vi "VRE17.vi"() -> ()   [LabVIEW 2012]
uses:
  <vilib>/userdefined/High Color/IMAQdx.ctl
  <vilib>/addons/Machine Learning/Utilities/Riffle (cluster).vi
  <vilib>/Analysis/baseanly.llb/Unimode.vi
  <vilib>/Analysis/baseanly.llb/Mean (DBL).vi
  <vilib>/Utility/file.llb/Write To Spreadsheet File (string).vi
  <vilib>/Utility/file.llb/Write To Spreadsheet File (DBL).vi
  <vilib>/regexp/Match Regular Expression.xnode
  <vilib>/vision/NI_Vision_Development_Module.lvlib
  <vilib>/vision/driver/NI_Vision_Acquisition_Software.lvlib
  <vilib>/Analysis/NI_AALBase.lvlib
  <vilib>/addons/Machine Learning/NILabs_MLT.lvlib
panel:
  in  "forced stop":bool
  out "Don't":bool
  out "LR invert all":bool
  in  "LR invert manual":bool
  out "moduleNum":u8
  out "moduleTime":u16
  out "nextMovieID":u8
  out "nextPerturbID":u8
  out "movieSeq":u8[](array[numeric])
  out "perturbSeq":u8[](array[numeric])
  in  "tON":u16=390
  in  "z3":u32=390
  in  "z1":u32=390
  out "moduleNumPrevious":u8
  out "moviePrimed":bool
  out "expTime":u16
  out "t0":u32
  out "movieR":u8
  out "active":i16
  out "m_buffer2":i8[](array[numeric])
  out "c_buffer 2":dbl[](array[numeric])
  out "w":dbl=50.0
  in  "Acquisition #":dbl
  in  "Basename":string
  out "sec":u16
  out "min":u16
  out "fileNumber":string
  in  "Tab Control":enum32{"User", "Manager", "protocol"}(tab)
  in  "Quiet mode":bool=TRUE
  in  "yawDrift":dbl=0.004
  in  "frdDrift":dbl=-0.002
  out "perturb wait":u16
  out "movie wait":u16
  out "perturb":u16(ring) items=["", "VR halt", "LR invert"]
  out "movie":u16(ring) items=["", "real fish", "h. ellipse", "v. ellipse", "feeding"]
  out "perturb ON":bool
  out "movie ON":bool
  out "movieID":u8
  out "perturbID":u8
  in  "LR invert":bool
  in  "yawCoef_L":dbl=1.1
  in  "yawCoef_R":dbl=1.1
  in  "keepSetting":bool
  in  "2P fps":dbl=30.0
  in  "Recording (min)":dbl=30.2
  out "2P frame":dbl
  in  "start experiment":bool
  in  "align done":bool
  out "LV loop time":u32
  in  "loop time (ms)":u32=20
  out "vreFps (ms)":dbl
  in  "frdCoef":dbl=0.25
  in  "yawIn threshold for movie":dbl=0.9
  in  "movie hijack":dbl=1.0
  in  "th1":dbl
  in  "th2":dbl
  out "m":dbl
  in  "Set baseline curv = 0 (for debug)":bool
  out "baseline curv":dbl
  in  "frdOmrVRE":bool
  in  "hijCoef2":dbl=10.0
  in  "hijCoef1":dbl=5.0
  in  "frd_hijack":dbl
  in  "yaw_hijack":i8
  in  "hijack":bool
  in  "th_darkBG":dbl=70.0
  out "blobs":dbl
  in  "decayR":dbl=0.9
  in  "cc^2":bool=TRUE
  in  "moviePrimedOff":u16=390
  in  "perturbDuration":u16=10
  in  "moviePrimedON":u16=240
  in  "perturbOnset":u16=120
  in  "modDuration":u16=450
  in  "Yres":i32=90
  in  "Xres":i32=120
  out "i":i32
  out "forward display":dbl(graph)
  in  "decayF":dbl=0.9
  out "zeroCross":i16
  out "cc":dbl
  out "m2":dbl[](array[numeric])
  out "m1":dbl[](array[numeric])
  out "I":u8[][](array[numeric])
  out "qCtr":dbl
  out "segL":dbl
  out "refine5ind":dbl[](array[numeric])
  out "xc":dbl
  out "yaw display":dbl(graph)
  out "cCurv1":dbl format="%0.2f"
  out "set 2P frames":dbl
  out "headingAngle":dbl
  out "virtual location":cluster{dbl[], dbl[]}[](graph)=[{[-0.0], [0.0]}, {[1.8369701987210297e-16], [3.0]}]
  out "trackPt":dbl[][](array[numeric])
  out "m_buffer":dbl[](array[numeric])
  out "c_buffer":dbl[](array[numeric])
  out "frdInput":dbl
  out "yawInput":dbl
  out "pix#":i32
  out "trackPt txt":path
  out "trackPt#":i32
  out "Image_save":T1(plugin-control) caption="Image"
  out "Session Out":T2
  out "data tif":refnum<file>
  in  "fx":dbl=120.0
  in  "fy":dbl=90.0
  out "par txt":path
  out "ROI":i32[](array[numeric])
  out "Bottom":i32
  out "Right":i32
  out "Top":i32
  out "Left":i32
  out "data txt":path
  out "y":dbl
  out "x":dbl
  out "forward":dbl
  out "yaw":dbl
  out "txt":dbl[][](array[numeric])
  out "txt row#":u64
  # "Right tunnel"
  # "Behavioral recording"
  # "27 min\n23 min\n18 min\n14 min\n10 min\n5 min\n1 min"
  # "Left tunnel"
  # "Set yawCoef_R & yawCoef_L so that max(yawInput) ~0.5"
  # "Set frdCoef so that max(frdInput) ~0.1"
  # "VRE update"
  # "VR perturbation"
  # "movie"
  # "VRE hijack"
  # "Define inactive frame to \nmeasure baseline curvature"
  # "Define active frames to \npermit classification"
  # "(in seconds)"
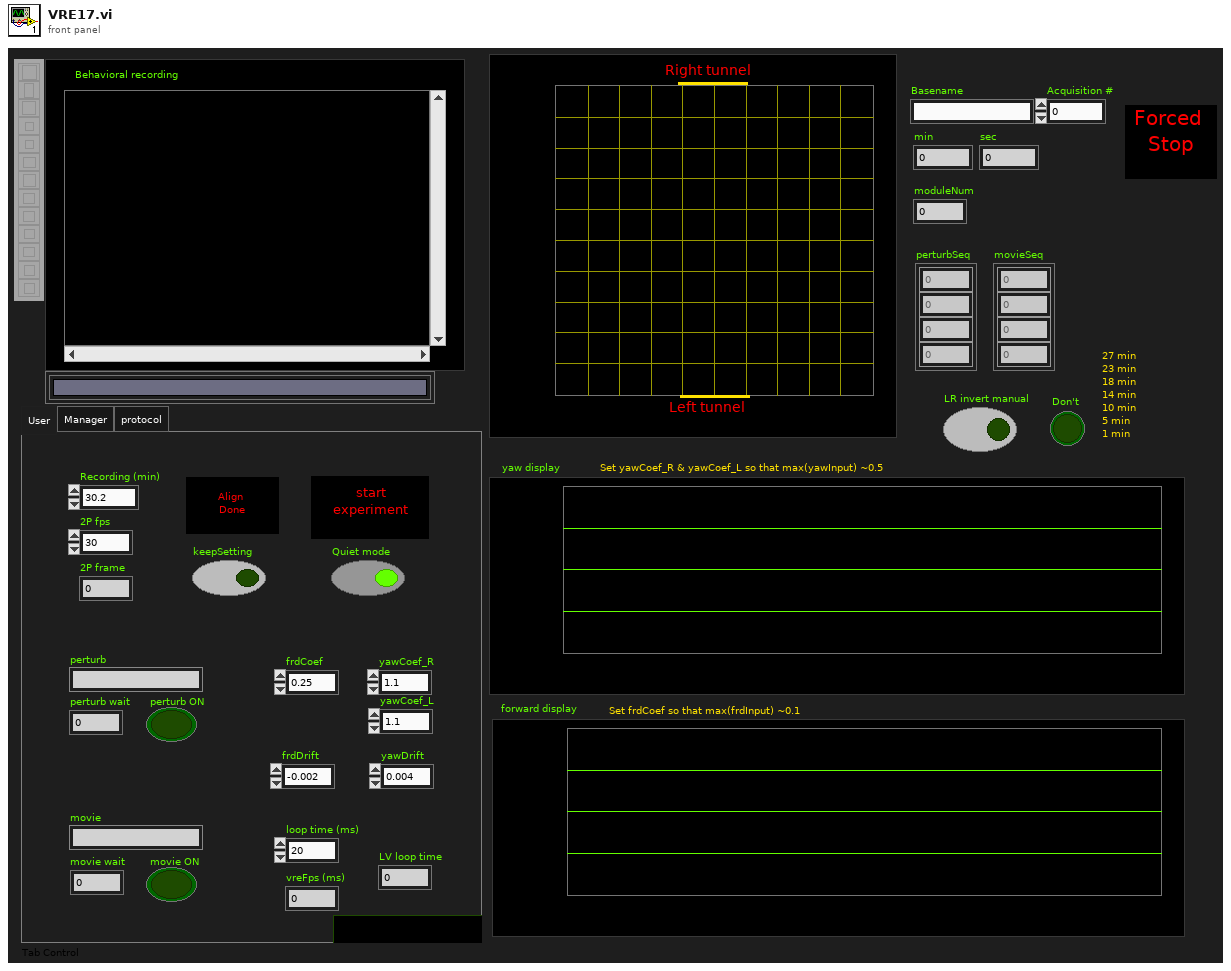
[diagram p1: front panel]
types:
  T1 = typedef "IMAQ Image.ctl" = refnum<image>
  T2 = typedef "IMAQdx.ctl" = refnum<k21>
  T3 = typedef "IMAQ Rectangle" = cluster{"Left":i32, "Top":i32, "Right":i32, "Bottom":i32, "Rotation":dbl}
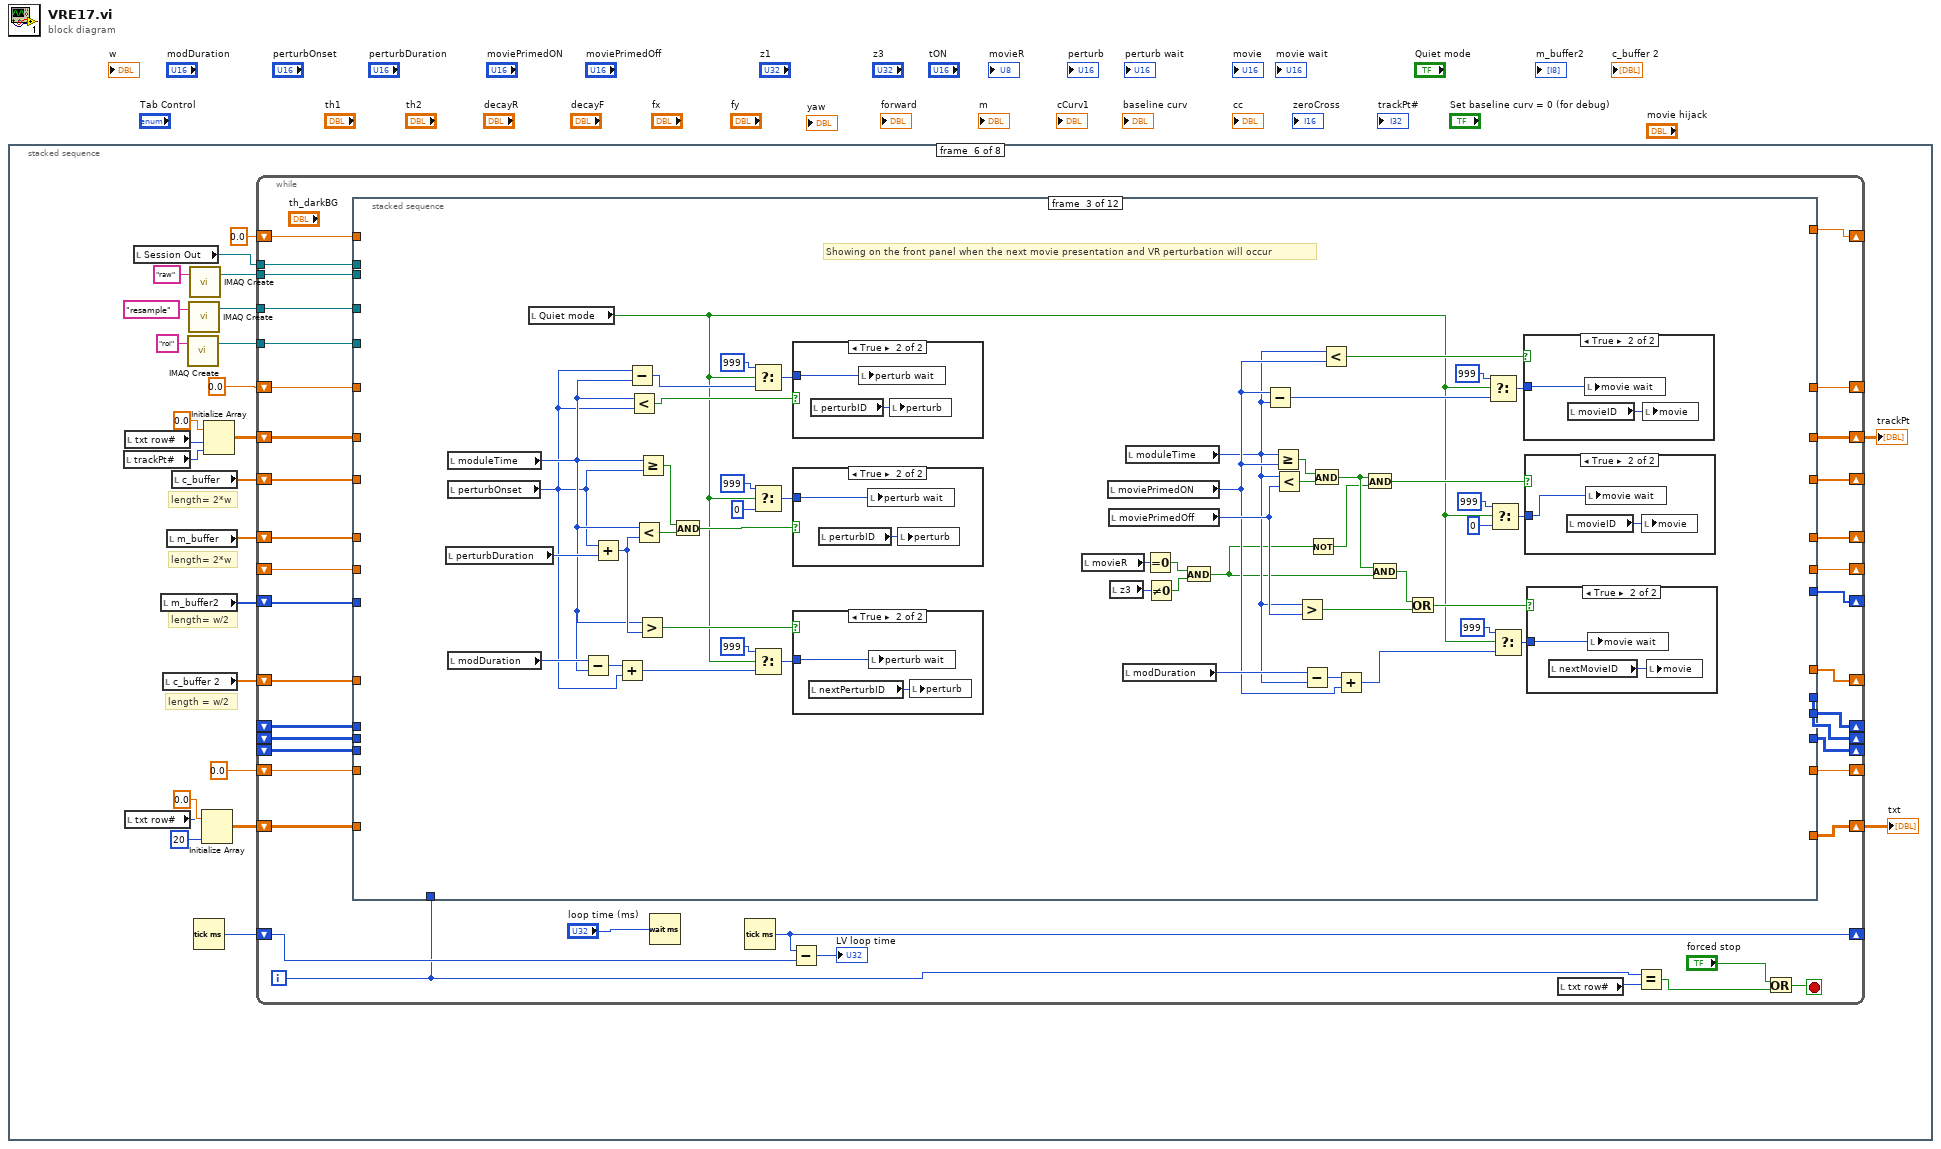
[diagram p0: block diagram]
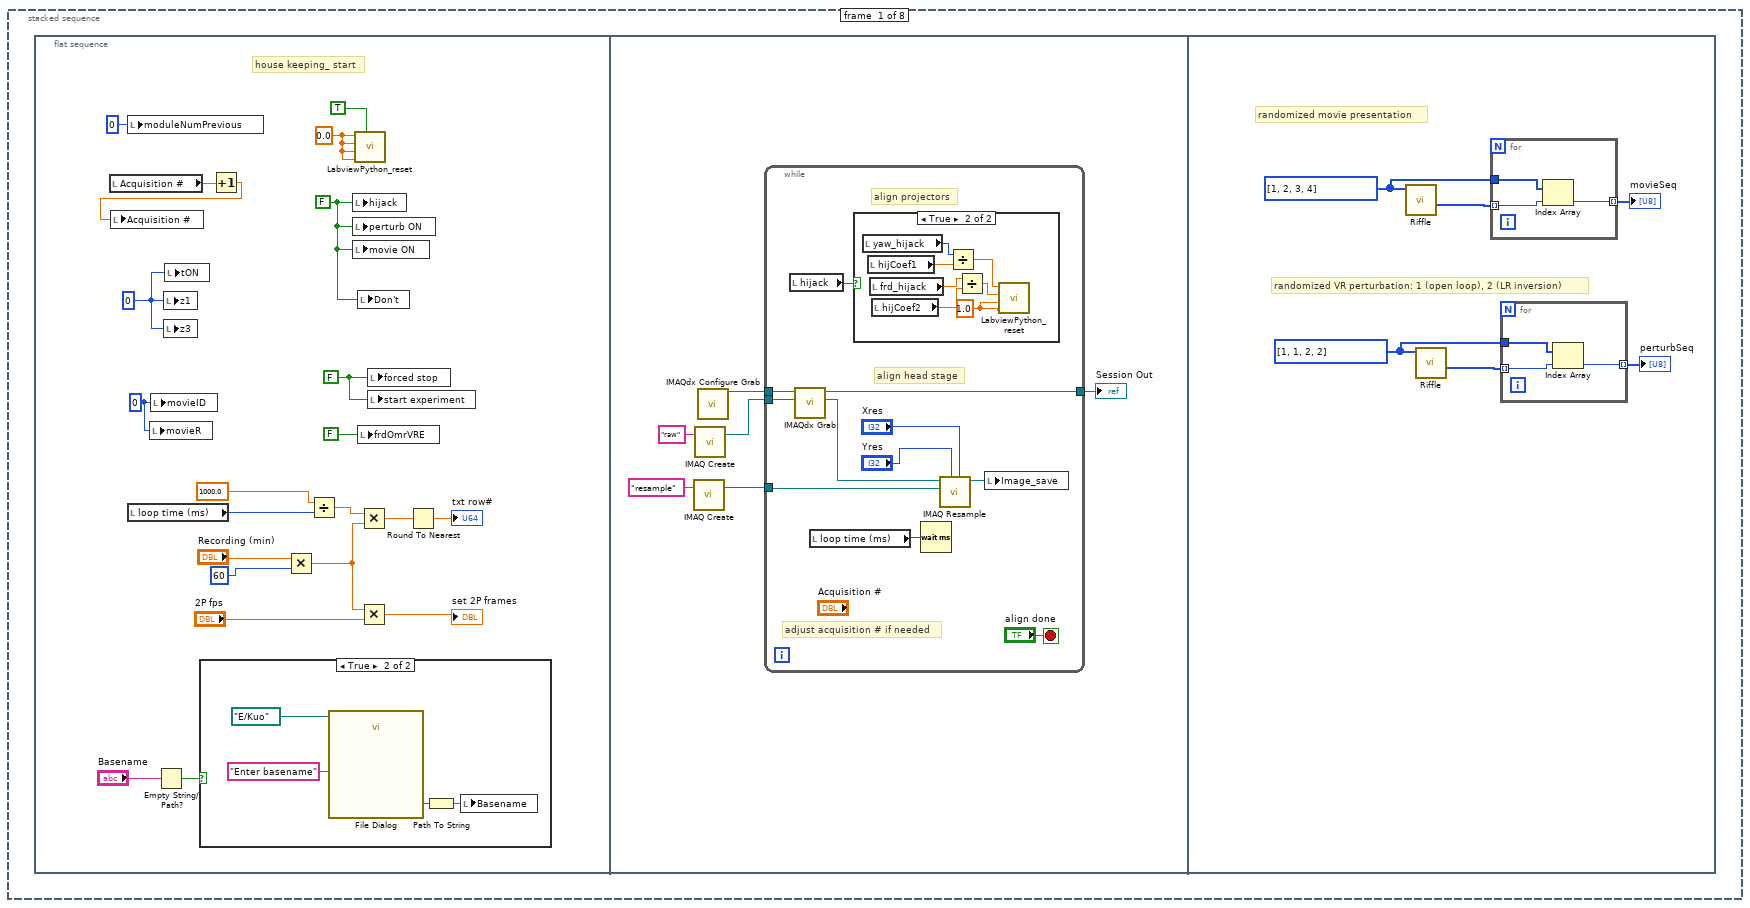
[diagram p2: hidden frame]
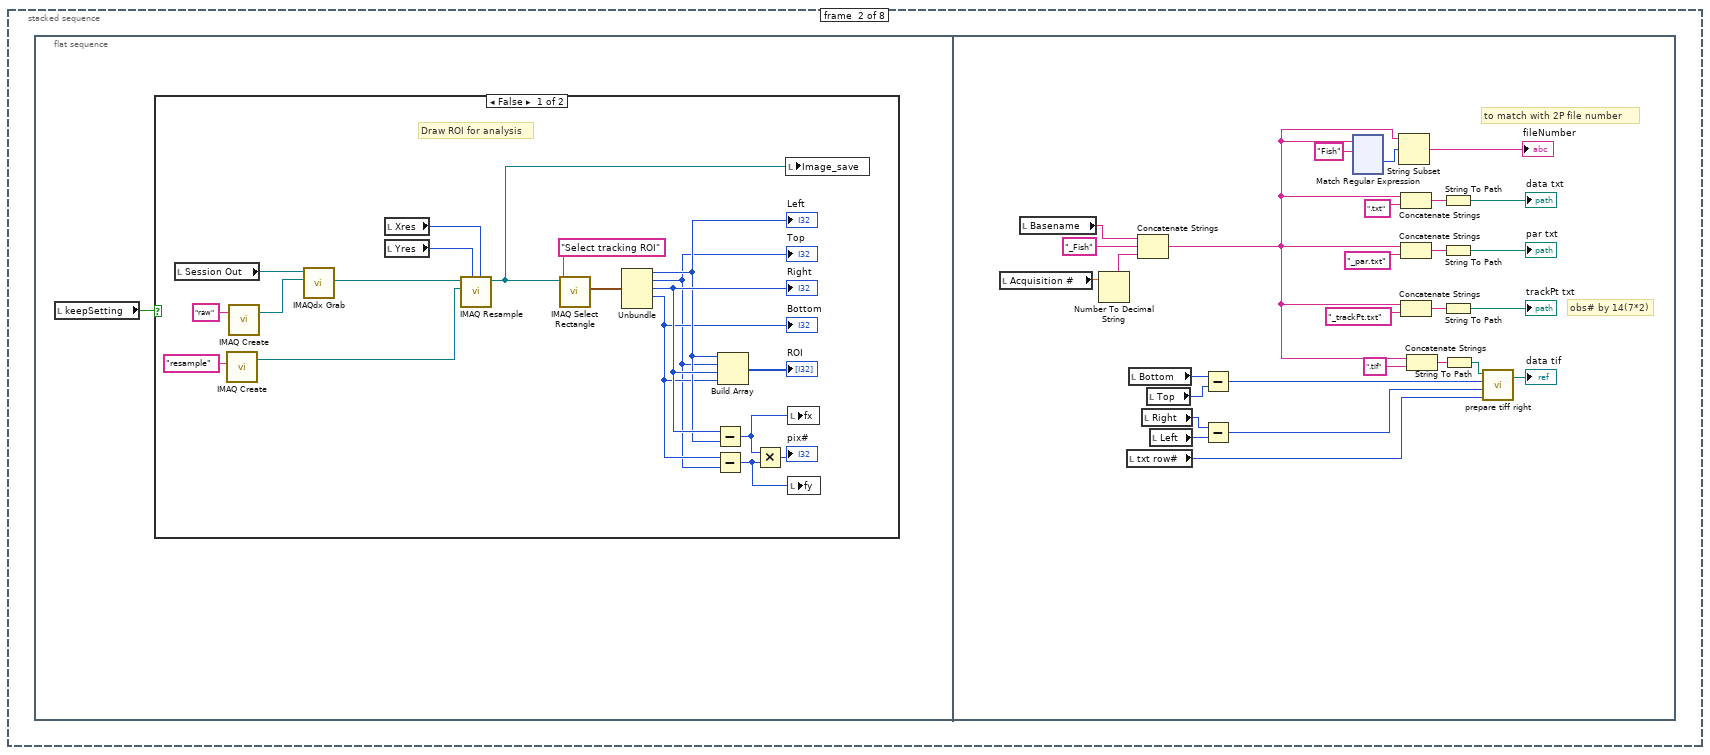
[diagram p5: hidden frame]
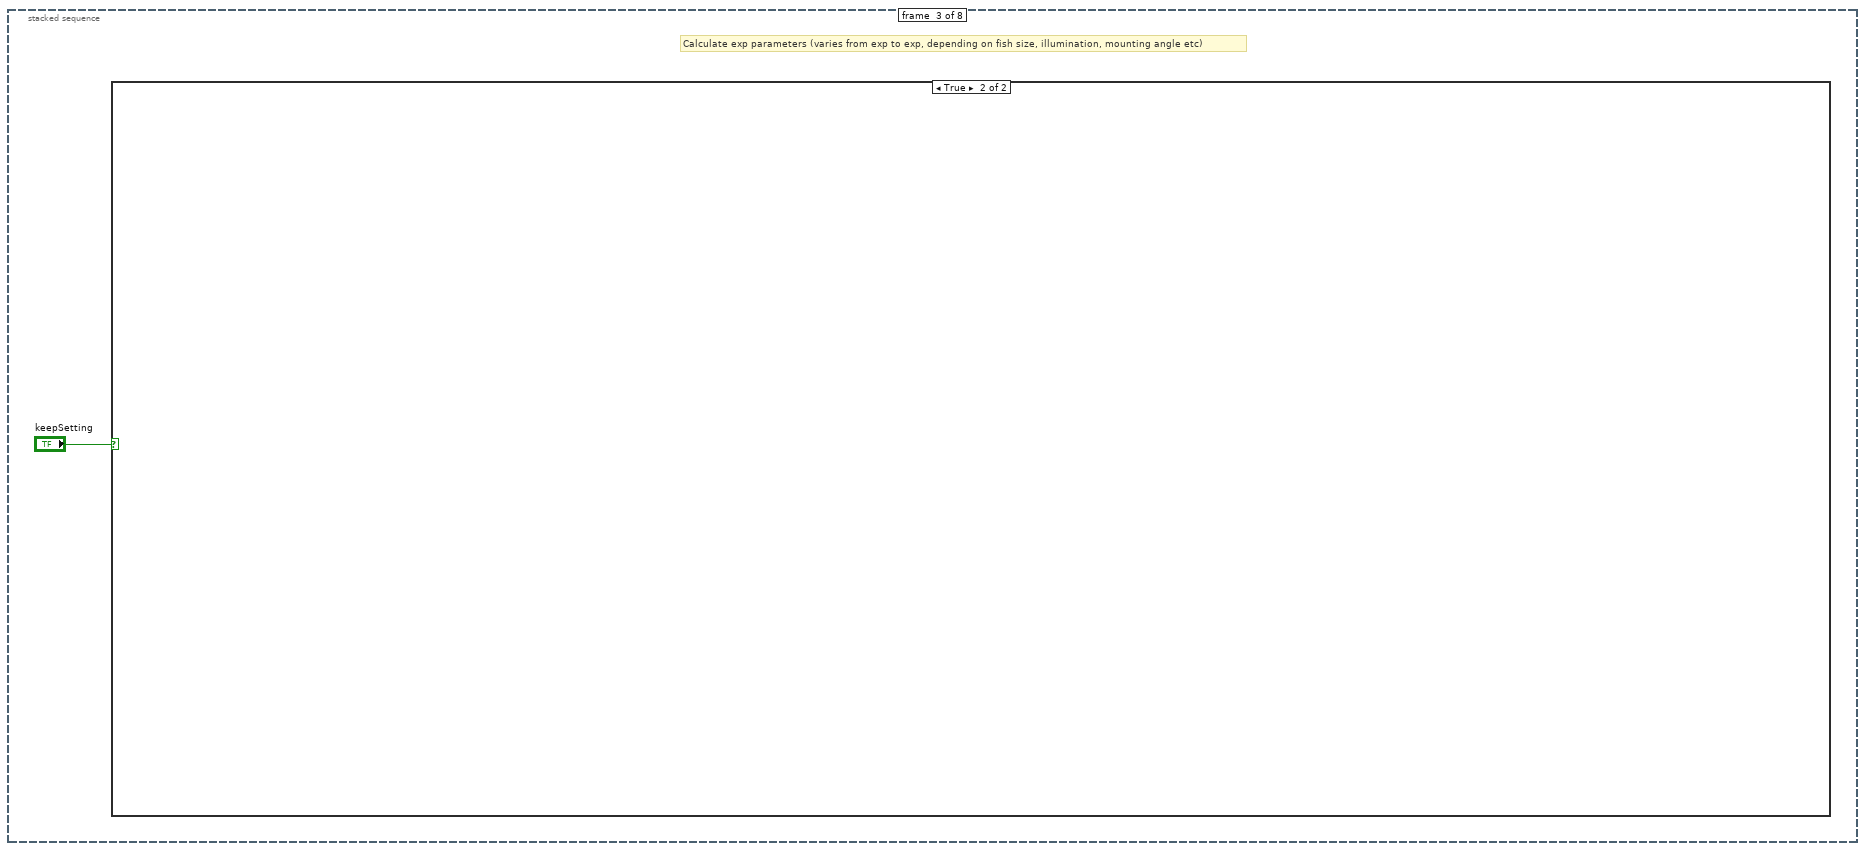
[diagram p7: hidden frame]
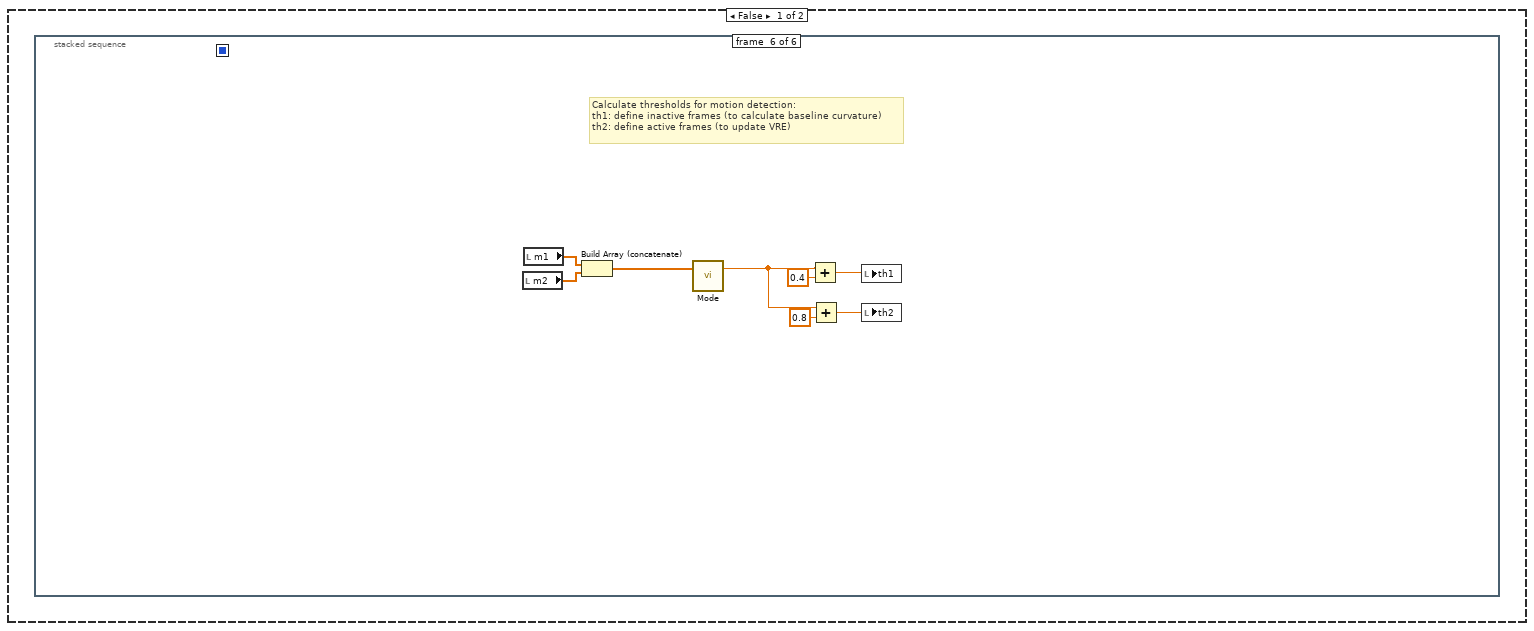
[diagram p8: hidden frame]
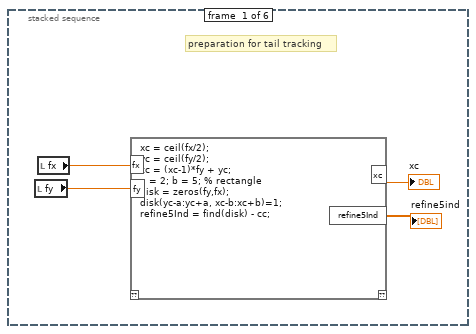
[diagram p9: hidden frame]
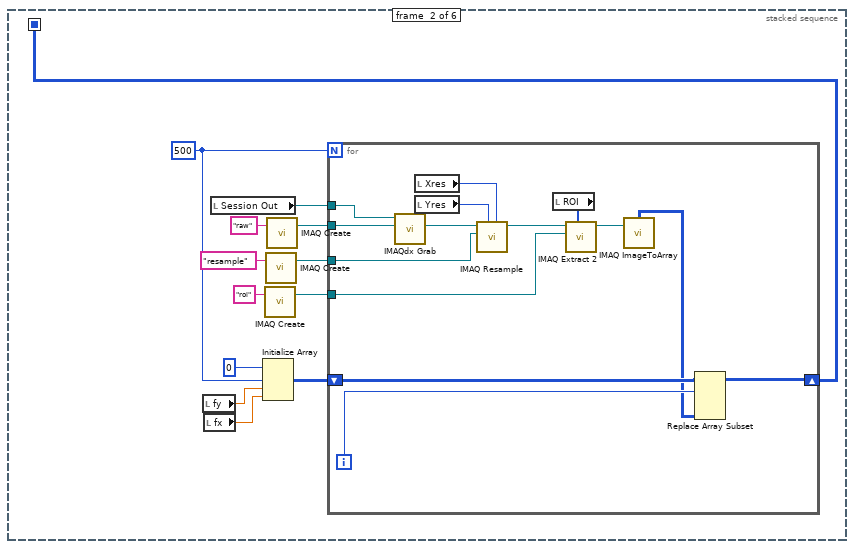
[diagram p10: hidden frame]
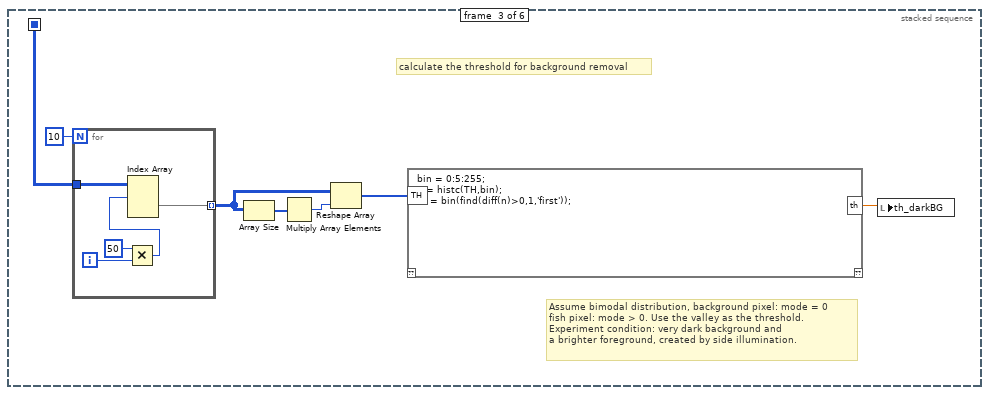
[diagram p11: hidden frame]
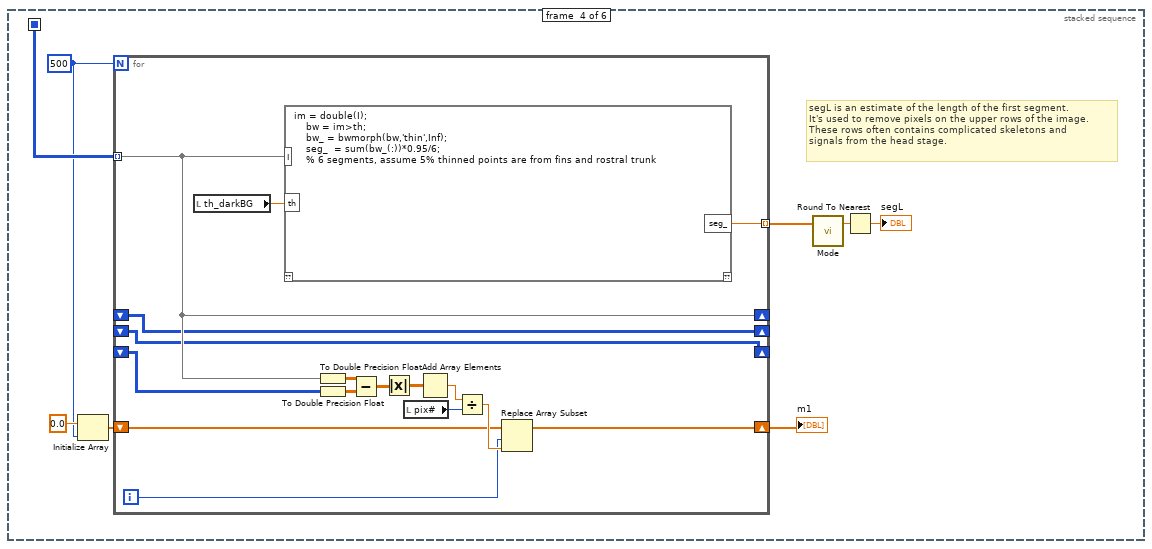
[diagram p12: hidden frame]
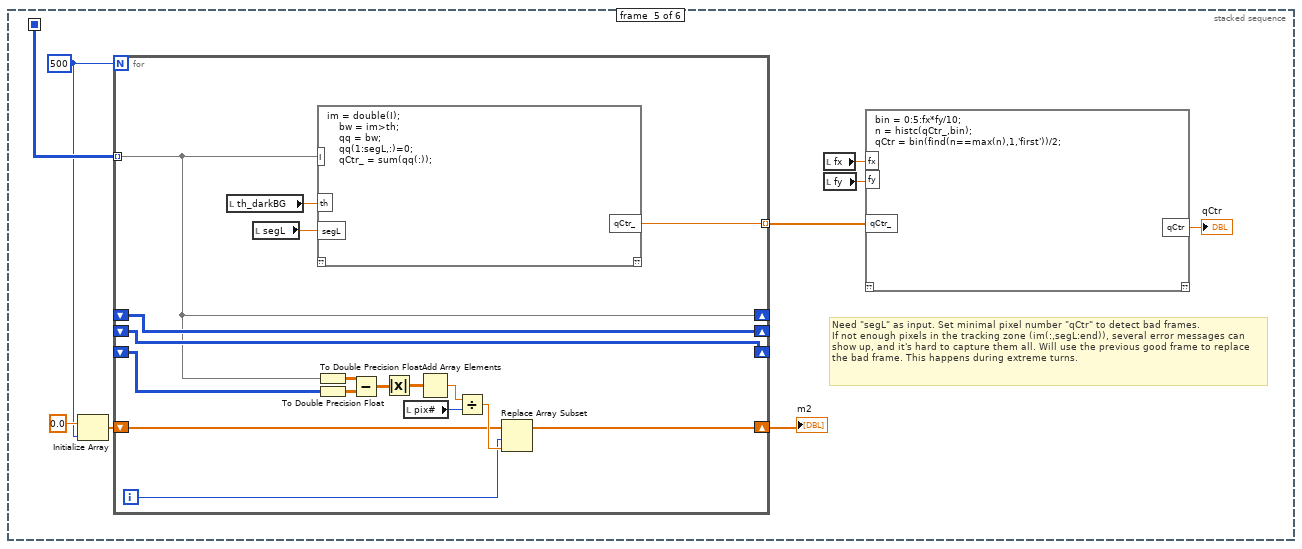
[diagram p13: hidden frame]
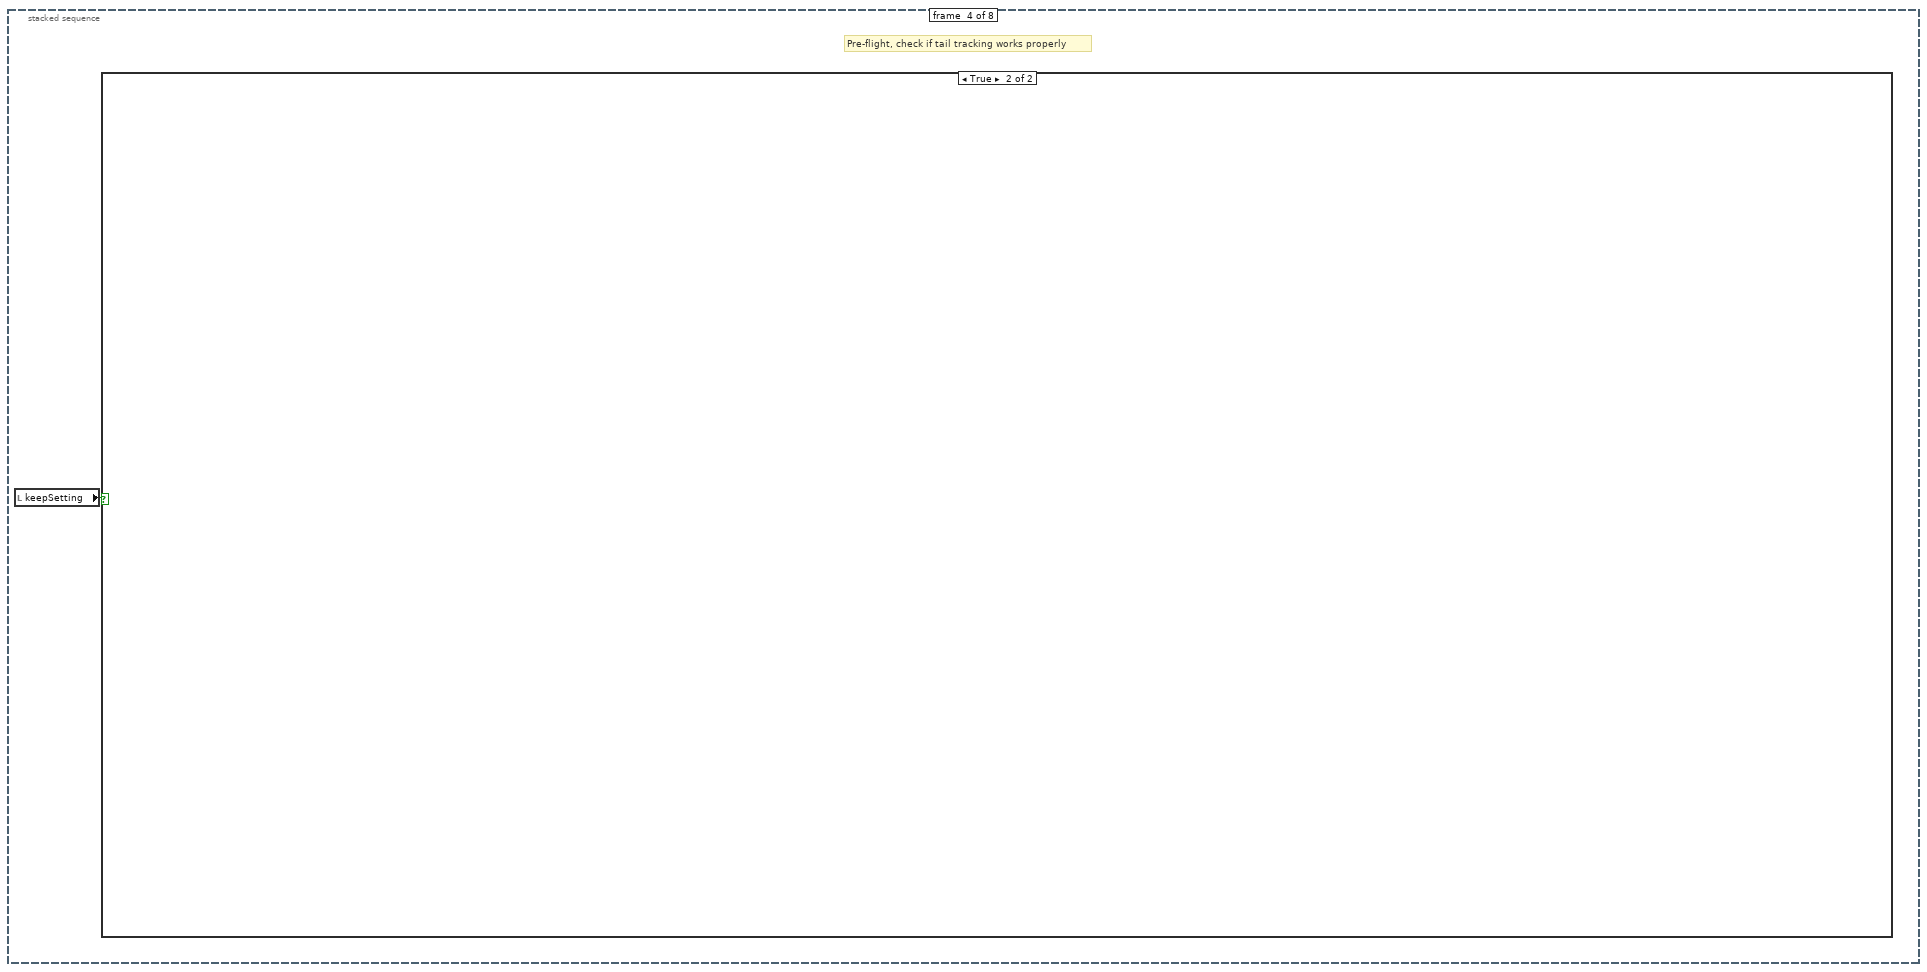
[diagram p14: hidden frame]
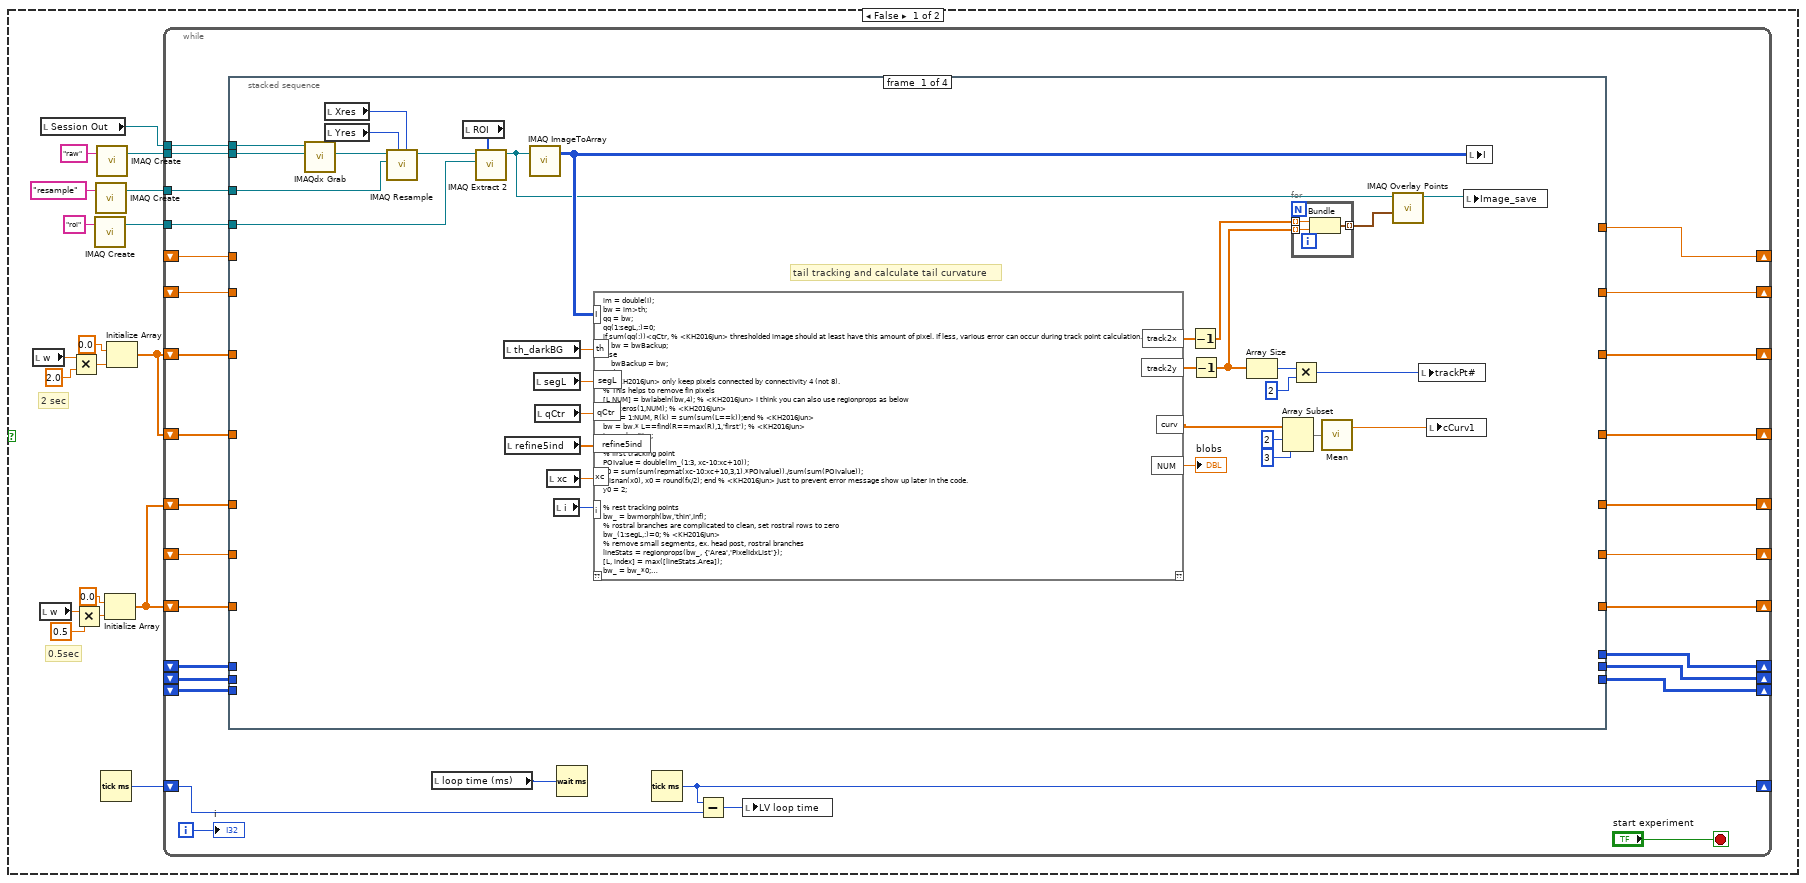
[diagram p15: hidden frame]
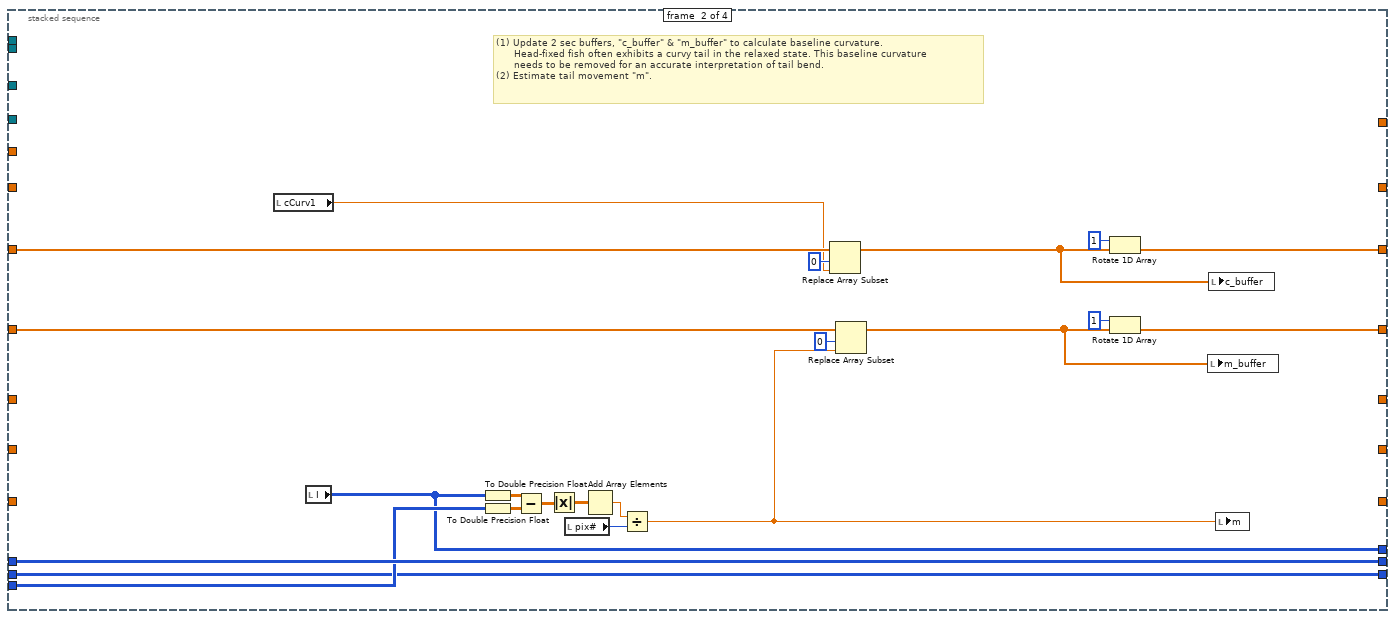
[diagram p16: hidden frame]
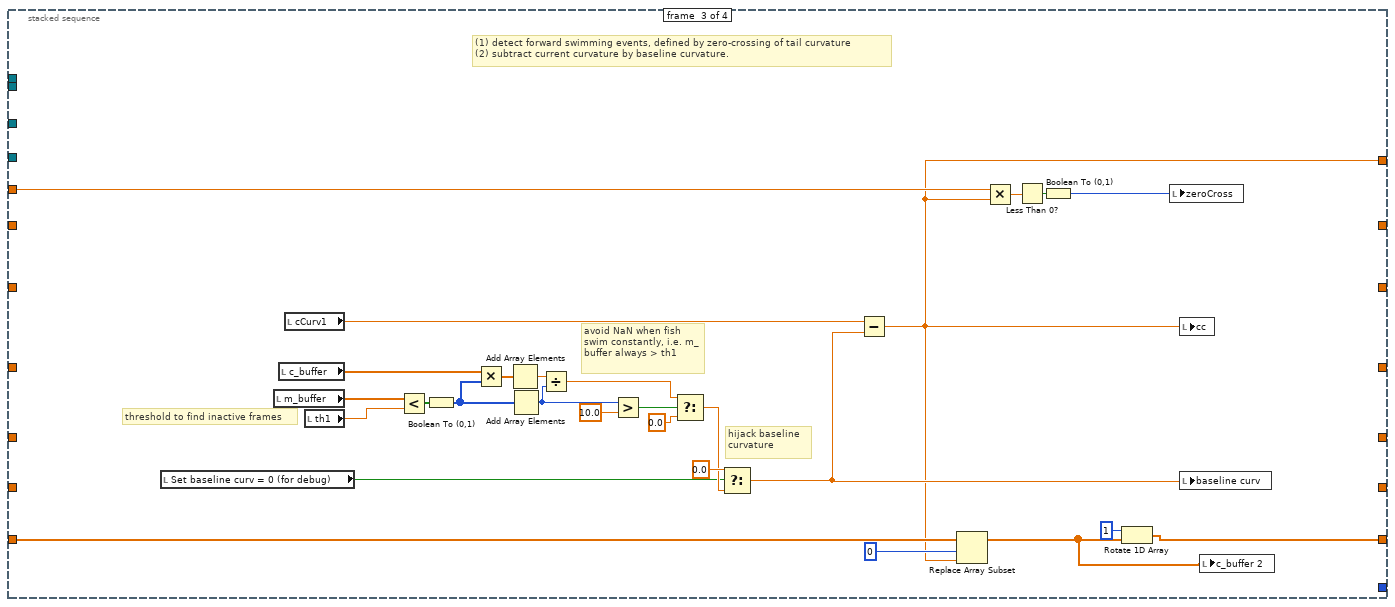
[diagram p17: hidden frame]
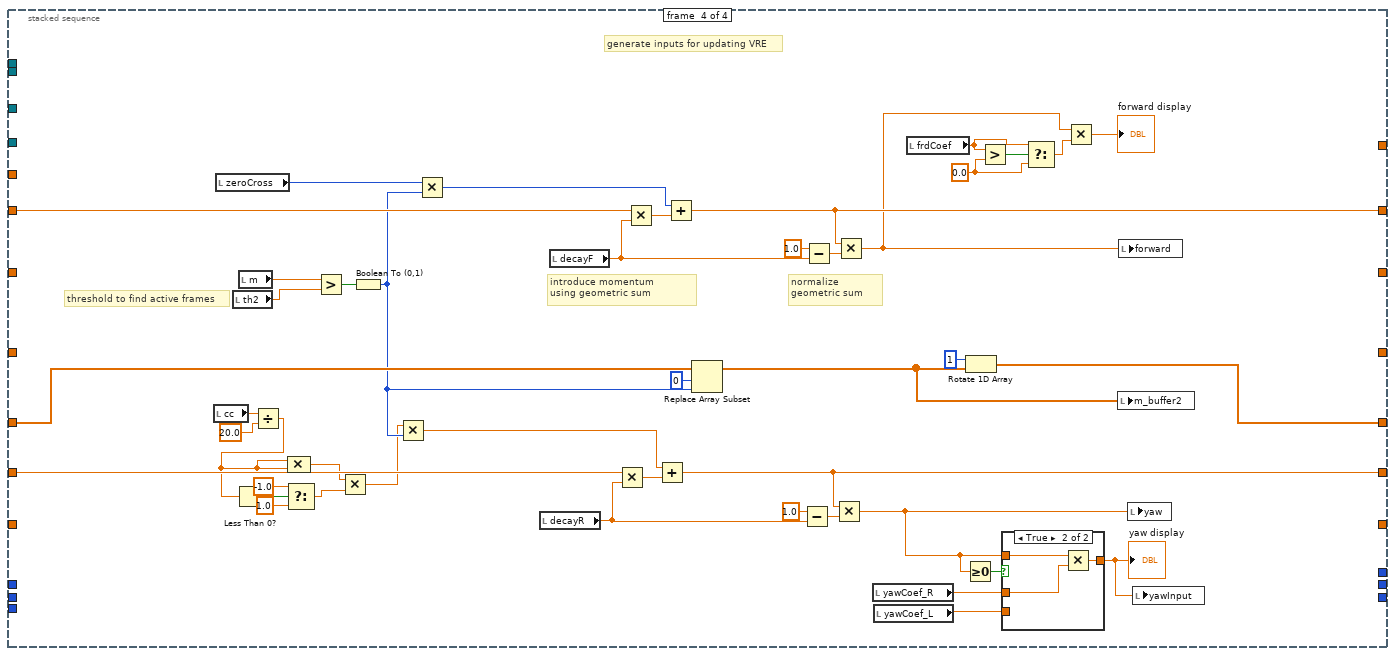
[diagram p18: hidden frame]
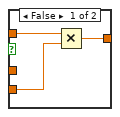
[diagram p19: hidden frame]
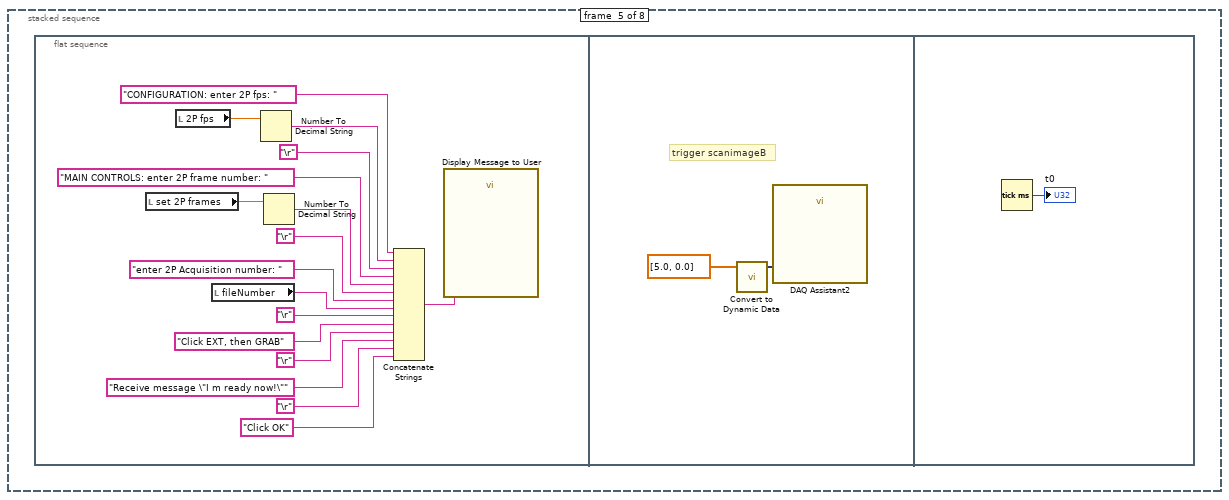
[diagram p20: hidden frame]
diagram:
  n1 = stacked-sequence {
    frame #0 {
      n2 = flat-sequence {
        frame #0 {
          w3 = u8 0 ("movieID")
          w2 = 0 ("z1")
          w1 = FALSE ("hijack")
          w19 = FALSE ("forced stop")
          w21 = 0.0 ("yaw_")
          # "house keeping_ start"
          n3 = local read "Acquisition #"() -> (w6:dbl)
          n4 = local write "moduleNumPrevious"(u8 0 ("moduleNumPrevious")) -> ()
          n5 = local read "loop time (ms)"() -> (w14:u32)
          n6 = local write "movieR"(w3) -> ()
          n7 = local write "movieID"(w3) -> ()
          n8 = Empty String/Path?(string/path="Basename") -> (empty?=w7:bool)
          n9 = local write "z1"(w2) -> ()
          n10 = local write "z3"(w2) -> ()
          n11 = local write "tON"(w2) -> ()
          n12 = case shown="True" w7 {
            frame False {
            }
            frame True {
              n13 = call "File Dialog"("start path"=path "E:/Kuo", "prompt"="Enter basename") -> ("selected path"=w25:path)  [unwired: 10 in, 3 out]
              n14 = Path To String(path=w25) -> (string=w26:string)
              n15 = local write "Basename"(w26) -> ()
            }
          }
          n16 = Increment(x=w6) -> (x+1=w5:dbl)
          n17 = local write "Acquisition #"(w5) -> ()
          n18 = Multiply(x="Recording (min)", y=u64 60) -> (x*y=w9:dbl)
          n19 = Divide(x=1000.0 ("y"), y=w14) -> (x/y=w11:dbl)
          n20 = local write "hijack"(w1) -> ()
          n21 = local write "perturb ON"(w1) -> ()
          n22 = local write "movie ON"(w1) -> ()
          n23 = call "LabviewPython_reset.vi"("reset_"=TRUE, "movie L"=w21, "movie R"=w21, "forward_"=w21, "yaw_"=w21) -> ()  [unwired: 3 in, 4 out]
          n24 = local write "Don't"(w1) -> ()
          n25 = local write "frdOmrVRE"(FALSE ("frdOmr")) -> ()
          n26 = Multiply(x=w11, y=w9) -> (x*y=w13:dbl)
          n27 = Multiply(x=w9, y="2P fps") -> (x*y=→"set 2P frames":dbl)
          n28 = local write "forced stop"(w19) -> ()
          n29 = local write "start experiment"(w19) -> ()
          n30 = Round To Nearest(number=w13) -> (nearest integer value=→"txt row#":dbl)
        }
        frame #1 {
          n31 = call "IMAQ Create"("Image Name"="resample") -> ("New Image"=w32:T1)  [unwired: 4 in, 1 out]
          n32 = call "IMAQ Create"("Image Name"="raw") -> ("New Image"=w29:T1)  [unwired: 4 in, 1 out]
          n33 = call <vilib>:"IMAQdx Configure Grab.vi"() -> ("Session Out"=w31:T2)  [unwired: 10 in, 1 out]
          n34 = while {
            tunnel: w31 -> [w43]
            tunnel: w29 -> [w42]
            tunnel: w32 -> [w39]
            tunnel: [w37] -> w27
            stop <- "align done" stop-if-true
            # "adjust acquisition # if needed"
            # "align projectors"
            # "align head stage"
            n35 = local read "hijack"() -> (w33:bool)
            n36 = call <vilib>:"IMAQdx Grab.vi"("Image In"=w42, "Session In"=w43) -> ("Image Out"=w40:T1, "Session Out"=w37:T2)  [unwired: 6 in, 2 out]
            n37 = local read "loop time (ms)"() -> (w34:u32)
            n38 = case shown="True" w33 {
              frame False {
              }
              frame True {
                w44 = 1.0 ("movie R")
                n39 = local read "yaw_hijack"() -> (w48:i8)
                n40 = local read "hijCoef1"() -> (w49:dbl)
                n41 = local read "frd_hijack"() -> (w47:dbl)
                n42 = local read "hijCoef2"() -> (w46:dbl)
                n43 = Divide(x=w48, y=w49) -> (x/y=w50:dbl)
                n44 = Divide(x=w47, y=w46) -> (x/y=w45:dbl)
                n45 = call "LabviewPython_reset.vi"("movie L"=w44, "movie R"=w44, "forward_"=w45, "yaw_"=w50) -> ()  [unwired: 4 in, 4 out]
              }
            }
            n46 = Wait (ms)(milliseconds to wait=w34) -> ()  [unwired: 1 out]
            n47 = call "IMAQ Resample"("X Resolution"="Xres", "Y Resolution"="Yres", "Image Dst"=w39, "Image Src"=w40) -> ("Image Dst Out"=w38:T1)  [unwired: 6 in, 1 out]
            n48 = local write "Image_save"(w38) -> ()
          }
          "Session Out" <- w27
        }
        frame #2 {
          w52 = u8[] [1, 1, 2, 2]
          w55 = u8[] [1, 2, 3, 4]
          # "randomized movie presentation"
          # "randomized VR perturbation: 1 (open loop), 2 (LR inversion)"
          n49 = call-poly <vilib>:"Riffle.vi"("Data samples"=w55) -> ("Riffled Index"=w56:i32[])  [unwired: 8 in, 2 out]
          n50 = call-poly <vilib>:"Riffle.vi"("Data samples"=w52) -> ("Riffled Index"=w51:i32[])  [unwired: 8 in, 2 out]
          n51 = for {
            tunnel: w56 -> [w62] mode=indexing
            tunnel: w55 -> [w61]
            tunnel: [w60] -> w54 mode=indexing
            n52 = Index Array(array=w61, index=w62) -> (element=w60:u8)
          }
          "movieSeq" <- w54
          n53 = for {
            tunnel: w51 -> [w59] mode=indexing
            tunnel: w52 -> [w58]
            tunnel: [w57] -> w53 mode=indexing
            n54 = Index Array(array=w58, index=w59) -> (element=w57:u8)
          }
          "perturbSeq" <- w53
        }
      }
    }
    frame #1 {
      n55 = flat-sequence {
        frame #0 {
          n56 = local read "keepSetting"() -> (w63:bool)
          n57 = case shown="False" w63 {
            frame False {
              # "Draw ROI for analysis"
              n58 = local read "Session Out"() -> (w80:T2)
              n59 = call "IMAQ Create"("Image Name"="resample") -> ("New Image"=w76:T1)  [unwired: 4 in, 1 out]
              n60 = call "IMAQ Create"("Image Name"="raw") -> ("New Image"=w79:T1)  [unwired: 4 in, 1 out]
              n61 = call <vilib>:"IMAQdx Grab.vi"("Image In"=w79, "Session In"=w80) -> ("Image Out"=w75:T1)  [unwired: 6 in, 3 out]
              n62 = local read "Xres"() -> (w67:i32)
              n63 = local read "Yres"() -> (w66:i32)
              n64 = call "IMAQ Resample"("X Resolution"=w67, "Y Resolution"=w66, "Image Dst"=w76, "Image Src"=w75) -> ("Image Dst Out"=w74:T1)  [unwired: 6 in, 1 out]
              n65 = call "IMAQ Select Rectangle"("Prompt"="Select tracking ROI", "Image In"=w74) -> ("Rectangle"=w81:T3)  [unwired: 6 in, 3 out]
              n66 = Unbundle(w81) -> ("Left"=w71:i32, "Top"=w69:i32, "Right"=w72:i32, "Bottom"=w70:i32)  [unwired: 1 out]
              "Left" <- w71
              "Top" <- w69
              "Right" <- w72
              "Bottom" <- w70
              n67 = Subtract(x=w72, y=w71) -> (x-y=w65:i32)
              n68 = Subtract(x=w70, y=w69) -> (x-y=w64:i32)
              n69 = Build Array(w71, w69, w72, w70) -> (→"ROI":i32[])
              n70 = Multiply(x=w65, y=w64) -> (x*y=→"pix#":i32)
              n71 = local write "Image_save"(w74) -> ()
              n72 = local write "fx"(w65) -> ()
              n73 = local write "fy"(w64) -> ()
            }
            frame True {
            }
          }
        }
        frame #1 {
          # "to match with 2P file number"
          # "obs# by 14(7*2)"
          n74 = local read "Acquisition #"() -> (w87:dbl)
          n75 = local read "Basename"() -> (w86:string)
          n76 = Number To Decimal String(number=w87) -> (decimal integer string=w84:string)  [unwired: 1 in]
          n77 = local read "txt row#"() -> (w91:u64)
          n78 = local read "Bottom"() -> (w92:i32)
          n79 = Concatenate Strings(w86, "_Fish" ("regular expression"), w84) -> (w83:string)
          n80 = local read "Right"() -> (w97:i32)
          n81 = local read "Top"() -> (w93:i32)
          n82 = local read "Left"() -> (w96:i32)
          n83 = Subtract(x=w92, y=w93) -> (x-y=w95:i32)
          n84 = Subtract(x=w97, y=w96) -> (x-y=w94:i32)
          n85 = xnode "Match Regular Expression"("input string"=w83, "regular expression"="Fish") -> ("offset past match"=w88:i32)  [unwired: 4 in, 4 out]
          n86 = String Subset(string=w83, offset (0)=w88) -> (substring=→"fileNumber":string)  [unwired: 1 in]
          n87 = Concatenate Strings(w83, ".txt") -> (w109:string)
          n88 = Concatenate Strings(w83, "_par.txt") -> (w106:string)
          n89 = Concatenate Strings(w83, "_trackPt.txt") -> (w103:string)
          n90 = Concatenate Strings(w83, ".tif" ("string")) -> (w100:string)
          n91 = String To Path(string=w109) -> (path=→"data txt":path)
          n92 = String To Path(string=w106) -> (path=→"par txt":path)
          n93 = String To Path(string=w103) -> (path=→"trackPt txt":path)
          n94 = String To Path(string=w100) -> (path=w99:path)
          n95 = call "prepare tiff right.vi"("z"=w91, "y"=w94, "x"=w95, "file path"=w99) -> ("refnum tif"=→"data tif":refnum<file>)  [unwired: 1 out]
        }
      }
    }
    frame #2 {
      # "Calculate exp parameters (varies from exp to exp, depending on fish size, illumination, mounting angle etc)"
      n96 = case shown="True" "keepSetting" {
        frame False {
          n97 = stacked-sequence {
            seq-local: [_ w227 _ _ _ _] -> [_ _ w256 w273 w298 _]
            frame #0 {
              # "preparation for tail tracking"
              n98 = local read "fy"() -> (w225:dbl)
              n99 = local read "fx"() -> (w226:dbl)
              n100 = script code="xc = ceil(fx/2);\nyc = ceil(fy/2);\ncc = (xc-1)*fy + yc;\na = 2; b = 5; % rectangle\ndisk = zeros(fy,fx);\ndisk(yc-a:yc+a, xc-b:xc+b)=1;\nrefine5Ind = find(disk) - cc;"("fx"=w226, "fy"=w225) -> ("xc"=→"xc":dbl, "refine5Ind"=→"refine5ind":dbl[])  [unwired: 1 in, 1 out]
            }
            frame #1 {
              w236 = 500 ("dimension size")
              n101 = local read "fy"() -> (w238:dbl)
              n102 = local read "fx"() -> (w237:dbl)
              n103 = local read "Session Out"() -> (w232:T2)
              n104 = Initialize Array(u8 0 ("element"), w236, w238, w237) -> (w228:u8[][][])
              n105 = call "IMAQ Create"("Image Name"="roi") -> ("New Image"=w229:T1)  [unwired: 4 in, 1 out]
              n106 = call "IMAQ Create"("Image Name"="resample") -> ("New Image"=w230:T1)  [unwired: 4 in, 1 out]
              n107 = call "IMAQ Create"("Image Name"="raw") -> ("New Image"=w231:T1)  [unwired: 4 in, 1 out]
              n108 = for {
                N: w236 -> [_]
                tunnel: w232 -> [w248]
                tunnel: w231 -> [w247]
                tunnel: w230 -> [w246]
                tunnel: w229 -> [w245]
                shift-right: [w243] -> w227
                shift-left: w228 -> [w244]
                i -> [w241]
                n109 = call <vilib>:"IMAQdx Grab.vi"("Image In"=w247, "Session In"=w248) -> ("Image Out"=w252:T1)  [unwired: 6 in, 3 out]
                n110 = local read "Xres"() -> (w249:i32)
                n111 = local read "Yres"() -> (w250:i32)
                n112 = call "IMAQ Resample"("X Resolution"=w249, "Y Resolution"=w250, "Image Dst"=w246, "Image Src"=w252) -> ("Image Dst Out"=w251:T1)  [unwired: 6 in, 1 out]
                n113 = local read "ROI"() -> (w253:i32[])
                n114 = call "IMAQ Extract 2"("Optional Rectangle"=w253, "Image Dst"=w245, "Image Src"=w251) -> ("Image Dst Out"=w242:T1)  [unwired: 7 in, 1 out]
                n115 = call "IMAQ ImageToArray"("Image"=w242) -> ("Image Pixels (U8)"=w240:u8[][])  [unwired: 3 in, 4 out]
                n116 = Replace Array Subset(array=w244, new element=w240, index (dim 0)=w241) -> (w243:u8[][][])  [unwired: 2 in]
              }
            }
            frame #2 {
              # "calculate the threshold for background removal"
              # "Assume bimodal distribution, background pixel: mode = 0\nfish pixel: mode > 0. Use the valley as the threshold.\nExperiment condition: very dark background and \na brighter foreground, created by side illumination."
              n117 = for {
                N: 10 -> [_]
                tunnel: w256 -> [w265]
                tunnel: [w261] -> w255 mode=indexing
                i -> [w264]
                n118 = Multiply(x=50 ("y"), y=w264) -> (x*y=w262:i32)
                n119 = Index Array(array=w265, index (dim 0)=w262) -> (element=w261:u8[][])  [unwired: 2 in]
              }
              n120 = Array Size(array=w255) -> (size(s)=w260:i32[])
              n121 = Multiply Array Elements(1:w260) -> (0:w259:i32)
              n122 = Reshape Array(w255, w259) -> (w258:u8[])
              n123 = script code="bin = 0:5:255;\nn = histc(TH,bin);\nth = bin(find(diff(n)>0,1,'first'));"("TH"=w258) -> ("th"=w254:dbl)  [unwired: 1 in, 1 out]
              n124 = local write "th_darkBG"(w254) -> ()
            }
            frame #3 {
              w268 = 500
              # "segL is an estimate of the length of the first segment. \nIt's used to remove pixels on the upper rows of the image. \nThese rows often contains complicated skeletons and \nsignals from the head stage."
              n125 = Initialize Array(0.0 ("element"), w268) -> (w267:dbl[])
              n126 = for {
                N: w268 -> [_]
                tunnel: w273 -> [w280] mode=indexing
                tunnel: [w289] -> w272 mode=indexing
                shift-right: [w280] -> _
                shift-left: _ -> [w279]
                shift-right: [w279] -> _
                shift-left: _ -> [w278]
                shift-right: [w278] -> _
                shift-left: _ -> [w277]
                shift-right: [w274] -> w266
                shift-left: w267 -> [w275]
                i -> [w281]
                n127 = local read "th_darkBG"() -> (w288:dbl)
                n128 = script code="im = double(I);    \n    bw = im>th;\n    bw_ = bwmorph(bw,'thin',Inf);\n    seg_  = sum(bw_(:))*0.95/6; \n    % 6 segments, assume 5% thinned points are from fins and rostral trunk"("I"=w280, "th"=w288) -> ("seg_"=w289:dbl)  [unwired: 1 in, 1 out]
                n129 = To Double Precision Float(number=w280) -> (double precision float=w283:dbl[][])
                n130 = To Double Precision Float(number=w277) -> (double precision float=w282:dbl[][])
                n131 = Subtract(x=w283, y=w282) -> (x-y=w287:dbl[][])
                n132 = Absolute Value(x=w287) -> (abs(x)=w286:dbl[][])
                n133 = local read "pix#"() -> (w276:i32)
                n134 = Add Array Elements(numeric array=w286) -> (sum=w285:dbl)
                n135 = Divide(x=w285, y=w276) -> (x/y=w284:dbl)
                n136 = Replace Array Subset(array=w275, new element=w284, index=w281) -> (w274:dbl[])
              }
              "m1" <- w266
              n137 = call-poly <vilib>:"Mode.vi"("X"=w272) -> ("mode"=w271:dbl)  [unwired: 1 in, 1 out]
              n138 = Round To Nearest(number=w271) -> (nearest integer value=→"segL":dbl)
            }
            frame #4 {
              w296 = 500
              # "Need \"segL\" as input. Set minimal pixel number \"qCtr\" to detect bad frames. \nIf not enough pixels in the tracking zone (im(:,segL:end)), several error messages can show up, and it's hard to capture them all. Will use the previous good frame to replace the bad frame. This happens during extreme turns."
              n139 = Initialize Array(0.0 ("element"), w296) -> (w295:dbl[])
              n140 = for {
                N: w296 -> [_]
                tunnel: w298 -> [w300] mode=indexing
                shift-right: [w300] -> _
                shift-left: _ -> [w308]
                shift-right: [w308] -> _
                shift-left: _ -> [w307]
                shift-right: [w307] -> _
                shift-left: _ -> [w306]
                shift-right: [w303] -> w294
                shift-left: w295 -> [w304]
                tunnel: [w299] -> w290 mode=indexing
                i -> [w309]
                n141 = local read "th_darkBG"() -> (w302:dbl)
                n142 = local read "segL"() -> (w301:dbl)
                n143 = script code="im = double(I);    \n    bw = im>th;\n    qq = bw;\n    qq(1:segL,:)=0; \n    qCtr_ = sum(qq(:));"("I"=w300, "th"=w302, "segL"=w301) -> ("qCtr_"=w299:dbl)  [unwired: 1 in, 1 out]
                n144 = To Double Precision Float(number=w300) -> (double precision float=w311:dbl[][])
                n145 = To Double Precision Float(number=w306) -> (double precision float=w310:dbl[][])
                n146 = Subtract(x=w311, y=w310) -> (x-y=w315:dbl[][])
                n147 = Absolute Value(x=w315) -> (abs(x)=w314:dbl[][])
                n148 = local read "pix#"() -> (w305:i32)
                n149 = Add Array Elements(numeric array=w314) -> (sum=w313:dbl)
                n150 = Divide(x=w313, y=w305) -> (x/y=w312:dbl)
                n151 = Replace Array Subset(array=w304, new element=w312, index=w309) -> (w303:dbl[])
              }
              "m2" <- w294
              n152 = local read "fx"() -> (w292:dbl)
              n153 = local read "fy"() -> (w293:dbl)
              n154 = script code="bin = 0:5:fx*fy/10;\nn = histc(qCtr_,bin);\nqCtr = bin(find(n==max(n),1,'first'))/2;"("fx"=w292, "qCtr_"=w290, "fy"=w293) -> ("qCtr"=→"qCtr":dbl)  [unwired: 1 in, 1 out]
            }
            frame #5 {
              # "Calculate thresholds for motion detection:\nth1: define inactive frames (to calculate baseline curvature)\nth2: define active frames (to update VRE)"
              n155 = local read "m2"() -> (w319:dbl[])
              n156 = local read "m1"() -> (w320:dbl[])
              n157 = Build Array (concatenate)(w320, w319) -> (w323:dbl[])
              n158 = call-poly <vilib>:"Mode.vi"("X"=w323) -> ("mode"=w317:dbl)  [unwired: 1 in, 1 out]
              n159 = Add(x=w317, y=0.4) -> (x+y=w321:dbl)
              n160 = Add(x=w317, y=0.8) -> (x+y=w318:dbl)
              n161 = local write "th1"(w321) -> ()
              n162 = local write "th2"(w318) -> ()
            }
          }
        }
        frame True {
        }
      }
    }
    frame #3 {
      # "Pre-flight, check if tail tracking works properly"
      n163 = local read "keepSetting"() -> (w324:bool)
      n164 = case shown="True" w324 {
        frame False {
          # "0.5sec"
          # "2 sec"
          n165 = local read "w"() -> (w330:dbl)
          n166 = local read "w"() -> (w331:dbl)
          n167 = local read "Session Out"() -> (w335:T2)
          n168 = Multiply(x=w330, y=2.0) -> (x*y=w328:dbl)
          n169 = Multiply(x=w331, y=0.5) -> (x*y=w327:dbl)
          n170 = call "IMAQ Create"("Image Name"="roi") -> ("New Image"=w339:T1)  [unwired: 4 in, 1 out]
          n171 = call "IMAQ Create"("Image Name"="resample") -> ("New Image"=w337:T1)  [unwired: 4 in, 1 out]
          n172 = call "IMAQ Create"("Image Name"="raw") -> ("New Image"=w341:T1)  [unwired: 4 in, 1 out]
          n173 = Tick Count (ms)() -> (millisecond timer value=w336:u32)
          n174 = Initialize Array(0.0 ("element"), w327) -> (w325:dbl[])
          n175 = Initialize Array(0.0 ("element"), w328) -> (w333:dbl[])
          n176 = while {
            tunnel: w341 -> [w372]
            shift-right: [w371] -> _
            shift-left: w336 -> [w370]
            tunnel: w339 -> [w369]
            tunnel: w337 -> [w368]
            tunnel: w335 -> [w367]
            shift-right: [w366] -> _
            shift-left: _ -> [w357]
            shift-right: [w360] -> _
            shift-left: _ -> [w359]
            shift-right: [w358] -> _
            shift-left: _ -> [w365]
            shift-right: [w361] -> _
            shift-left: w333 -> [w364]
            shift-right: [w362] -> _
            shift-left: w333 -> [w363]
            shift-right: [w353] -> _
            shift-left: _ -> [w350]
            shift-right: [w351] -> _
            shift-left: _ -> [w352]
            shift-right: [w348] -> _
            shift-left: _ -> [w349]
            shift-right: [w343] -> _
            shift-left: w325 -> [w346]
            shift-right: [w344] -> _
            shift-left: w325 -> [w345]
            i -> [w347]
            stop <- "start experiment" stop-if-true
            n177 = stacked-sequence {
              tunnel: w372 -> [w404 _ _ _]
              tunnel: w369 -> [w403 _ _ _]
              tunnel: w368 -> [w402 _ _ _]
              tunnel: w367 -> [w401 _ _ _]
              tunnel: [_ w408 _ _] -> w366
              tunnel: w365 -> [_ w414 _ _]
              tunnel: w364 -> [_ w429 _ _]
              tunnel: w363 -> [_ w418 _ _]
              tunnel: [_ w417 _ _] -> w362
              tunnel: [_ w416 _ _] -> w361
              tunnel: [_ w415 _ _] -> w360
              tunnel: w359 -> [_ w413 _ _]
              tunnel: [_ w413 _ _] -> w358
              tunnel: w357 -> [_ w415 _ _]
              tunnel: [_ _ w432 _] -> w353
              tunnel: w352 -> [_ _ _ w493]
              tunnel: [_ _ _ w491] -> w351
              tunnel: w350 -> [_ _ w439 _]
              tunnel: w349 -> [_ _ _ w488]
              tunnel: [_ _ _ w483] -> w348
              tunnel: w346 -> [_ _ w433 _]
              tunnel: w345 -> [_ _ _ w480]
              tunnel: [_ _ _ w478] -> w344
              tunnel: [_ _ w430 _] -> w343
              frame #0 {
                # "tail tracking and calculate tail curvature"
                n178 = call <vilib>:"IMAQdx Grab.vi"("Image In"=w404, "Session In"=w401) -> ("Image Out"=w399:T1)  [unwired: 6 in, 3 out]
                n179 = local read "Xres"() -> (w393:i32)
                n180 = local read "Yres"() -> (w394:i32)
                n181 = call "IMAQ Resample"("X Resolution"=w393, "Y Resolution"=w394, "Image Dst"=w402, "Image Src"=w399) -> ("Image Dst Out"=w398:T1)  [unwired: 6 in, 1 out]
                n182 = local read "ROI"() -> (w400:i32[])
                n183 = call "IMAQ Extract 2"("Optional Rectangle"=w400, "Image Dst"=w403, "Image Src"=w398) -> ("Image Dst Out"=w374:T1)  [unwired: 7 in, 1 out]
                n184 = local read "th_darkBG"() -> (w386:dbl)
                n185 = local read "refine5ind"() -> (w389:dbl[])
                n186 = call "IMAQ ImageToArray"("Image"=w374) -> ("Image Pixels (U8)"=w379:u8[][])  [unwired: 3 in, 4 out]
                n187 = local read "segL"() -> (w387:dbl)
                n188 = local read "qCtr"() -> (w388:dbl)
                n189 = local read "xc"() -> (w390:dbl)
                n190 = local read "i"() -> (w380:i32)
                n191 = script code="im = double(I);\nbw = im>th;\nqq = bw;\nqq(1:segL,:)=0;\nif sum(qq(:))<qCtr, % <KH2016Jun> thresholded image should at least have this amount of pixel. If less, various error can occur during track point calculation.\n    bw = bwBackup;\nelse\n    bwBackup = bw;\nend\n% <KH2016Jun> only keep pixels connected by connectivity 4 (not 8).\n% This helps to remove fin pixels\n[L NUM] = bwlabeln(bw,4); % <KH2016Jun> I think you can also use regionprops as below\nR = zeros(1,NUM); % <KH2016Jun>\nfor k = 1:NUM, R(k) = sum(sum(L==k));end % <KH2016Jun>\nbw = bw.* L==find(R==max(R),1,'first'); % <KH2016Jun>\nim_ = bw.*im;\n\n% first tracking point\nPOIvalue = double(im_(1:3, xc-10:xc+10));\nx0 = sum(sum(repmat(xc-10:xc+10,3,1).*POIvalue))./sum(sum(POIvalue));\nif isnan(x0), x0 = round(fx/2); end % <KH2016Jun> Just to prevent error message show up later in the code.\ny0 = 2;\n\n% rest tracking points\nbw_ = bwmorph(bw,'thin',Inf);\n% rostral branches are complicated to clean, set rostral rows to zero\nbw_(1:segL,:)=0; % <KH2016Jun>\n% remove small segments, ex. head post, rostral branches\nlineStats = regionprops(bw_, {'Area','PixelIdxList'});\n[L, index] = max([lineStats.Area]);\nbw_ = bw_*0;\nbw_(lineStats(index).PixelIdxList) = 1;\n\nc = sum(bw_(:));\nind = find(bw_);\nPOI = repmat(refine5Ind,1,c)+repmat(ind',length(refine5Ind),1);\nif sum(sum(POI>(size(bw,1)*size(bw,2)) | POI<1))~= 0 % <KH2016Jun> In case POI is out of image range\n    POI = ones(size(POI));\nend\n\nPOIx = ceil(POI/fy);\nPOIy = rem(POI,fy);\nPOIvalue = double(im_(POI));\nx_ = sum(POIx.*POIvalue)./sum(POIvalue);\ny_ = sum(POIy.*POIvalue)./sum(POIvalue);\ntrackA = [x0, x_; y0, y_]; % non-sorted track points\n\nseed = [x0;y0];\nseedInd = 1;\ntrack_ = [zeros(2,1) trackA(:,2:end)]; % temporary registry\ntrack = trackA; % to store sorted track points\nfor j = 1:size(track,2)-1\n    d = ((track_(1,:)-seed(1)).^2 + (track_(2,:)-seed(2)).^2); % distance of all remaining points to the seed\n    targetInd = find(d==min(d),1,'first');\n    target = track_(:, targetInd);\n    track(:,j+1) = target;\n    seed = target;\n    track_(:,targetInd)=0;\nend\n\n% cut tail into 6 segments, (x0,y0)>(x1, y1) is seg 1. (x1, y1) > (xn, yn) is cut to 5 segments\nsegSize = (size(track,2)-2)/5; % an estimate of segment length (# of track point).\n% segSize is similar to segL, but it's more precise. IMP: do not try to replace with segL.\nt2 = track(:,round(2:segSize:size(track,2)));\nd2 = mean(sum(diff(t2,1,2).^2)); % an estimate of segment length (pixel distance)\ntrack_ = track(:,2:end-1); %<KH2016Jun>\nseed  = track_(:,1);\ntrack2 = [track(:,1:2) zeros(2,4) track(:,end)];\nfor j = 1:4\n    d = abs(((track_(1,:)-seed(1)).^2 + (track_(2,:)-seed(2)).^2)-d2);\n    targetInd = find(d==min(d),1,'first');\n    target = track_(:, targetInd);\n    track2(:,j+2) = target;\n    seed = target;\n    track_(:,1:targetInd)=0;\nend\n\ndV = diff(track2,[],2);\nAngle = atan(dV(1,:) ./ dV(2,:))/pi*180; % -90<angle<90\n% expand Angle from -90<angle<90 to -180<angle< 180\nAngle(dV(2,:)<0) = Angle(dV(2,:)<0) +180; %<KH2016Jun> -90<angle<270\nAngle(Angle>180) = Angle(Angle>180) -360; %<KH2016Jun> -180<angle<180\ncurv = diff(Angle);\n\ndd = sqrt(sum(diff(track2,1,2).^2));\nif sum(abs(curv)>60)==0 && sum(isnan(curv))==0 && sum(dd<segSize*0.5)==0%<KH2016Jun>\n    track2backup = track2;\n    curvBackup = curv;\nelse\n    if i==0;\n        track2 = [fx/2*ones(1,7);1:5:31]; % if first frame is bad, just set it as a vertical straight line\n        curv = zeros(1,5);\n    else\n        track2 = track2backup;\n        curv = curvBackup;\n    end\nend\n\ntrack2x = track2(1,:);\ntrack2y = track2(2,:);" ("Script Node")("I"=w379, "th"=w386, "segL"=w387, "qCtr"=w388, "refine5ind"=w389, "xc"=w390, "i"=w380) -> ("track2x"=w385:dbl[], "track2y"=w384:dbl[], "curv"=w383:dbl[], "NUM"=→"blobs":dbl)  [unwired: 1 in, 1 out]
                n192 = Decrement(x=w385) -> (x-1=w376:dbl[])
                n193 = Decrement(x=w384) -> (x-1=w375:dbl[])
                n194 = Array Size(array=w375) -> (size(s)=w392:i32)
                n195 = Array Subset(array=w383, index=2, length=3) -> (w395:dbl[])
                n196 = Multiply(x=w392, y=2) -> (x*y=w382:i32)
                n197 = for {
                  tunnel: w376 -> [w407] mode=indexing
                  tunnel: w375 -> [w406] mode=indexing
                  tunnel: [w405] -> w378 mode=indexing
                  n198 = Bundle(w407, w406) -> (w405:cluster{dbl, dbl})  [unwired: 1 in]
                }
                n199 = call-poly <vilib>:"Mean.vi"("X"=w395) -> ("mean"=w381:dbl)  [unwired: 1 out]
                n200 = call "IMAQ Overlay Points"("Array of Points"=w378, "Image"=w374) -> ("Image Out"=w377:T1)  [unwired: 8 in, 1 out]
                n201 = local write "trackPt#"(w382) -> ()
                n202 = local write "cCurv1"(w381) -> ()
                n203 = local write "Image_save"(w377) -> ()
                n204 = local write "I"(w379) -> ()
              }
              frame #1 {
                # "(1) Update 2 sec buffers, \"c_buffer\" & \"m_buffer\" to calculate baseline curvature.\n      Head-fixed fish often exhibits a curvy tail in the relaxed state. This baseline curvature      \n      needs to be removed for an accurate interpretation of tail bend.\n(2) Estimate tail movement \"m\"."
                n205 = local read "cCurv1"() -> (w412:dbl)
                n206 = local read "I"() -> (w408:u8[][])
                n207 = To Double Precision Float(number=w408) -> (double precision float=w425:dbl[][])
                n208 = To Double Precision Float(number=w414) -> (double precision float=w424:dbl[][])
                n209 = Subtract(x=w425, y=w424) -> (x-y=w428:dbl[][])
                n210 = Absolute Value(x=w428) -> (abs(x)=w427:dbl[][])
                n211 = local read "pix#"() -> (w423:i32)
                n212 = Add Array Elements(numeric array=w427) -> (sum=w426:dbl)
                n213 = Divide(x=w426, y=w423) -> (x/y=w409:dbl)
                n214 = Replace Array Subset(array=w429, new element=w412, index=0) -> (w411:dbl[])
                n215 = Replace Array Subset(array=w418, new element=w409, index=0) -> (w410:dbl[])
                n216 = Rotate 1D Array(1:w411, 2:1 ("n")) -> (0:w416:dbl[])
                n217 = Rotate 1D Array(1:w410, 2:1 ("n")) -> (0:w417:dbl[])
                n218 = local write "m_buffer"(w410) -> ()
                n219 = local write "c_buffer"(w411) -> ()
                n220 = local write "m"(w409) -> ()
              }
              frame #2 {
                # "avoid NaN when fish swim constantly, i.e. m_buffer always > th1"
                # "hijack baseline curvature"
                # "(1) detect forward swimming events, defined by zero-crossing of tail curvature \n(2) subtract current curvature by baseline curvature."
                # "threshold to find inactive frames"
                n221 = local read "Set baseline curv = 0 (for debug)"() -> (w436:bool)
                n222 = local read "m_buffer"() -> (w450:dbl[])
                n223 = local read "c_buffer"() -> (w451:dbl[])
                n224 = local read "cCurv1"() -> (w449:dbl)
                n225 = local read "th1"() -> (w453:dbl)
                n226 = Less?(x=w450, y=w453) -> (x < y?=w454:bool[])
                n227 = Boolean To (0,1)(Boolean=w454) -> (0, 1=w456:i16[])
                n228 = Multiply(x=w451, y=w456) -> (x*y=w455:dbl[])
                n229 = Add Array Elements(numeric array=w455) -> (sum=w452:dbl)
                n230 = Add Array Elements(numeric array=w456) -> (sum=w442:i16)
                n231 = Divide(x=w452, y=w442) -> (x/y=w443:dbl)
                n232 = Greater?(x=w442, y=10.0) -> (0:w445:bool)
                n233 = Select(t=w443, s=w445, f=0.0) -> (s? t:f=w447:dbl)
                n234 = Select(t=0.0, s=w436, f=w447) -> (s? t:f=w438:dbl)
                n235 = Subtract(x=w449, y=w438) -> (x-y=w432:dbl)
                n236 = Replace Array Subset(array=w433, new element=w432, index=0) -> (w431:dbl[])
                n237 = Multiply(x=w439, y=w432) -> (x*y=w440:dbl)
                n238 = Less Than 0?(x=w440) -> (x < 0?=w441:bool)
                n239 = Boolean To (0,1)(Boolean=w441) -> (0, 1=w437:i16)
                n240 = Rotate 1D Array(1:w431, 2:1 ("n")) -> (0:w430:dbl[])
                n241 = local write "zeroCross"(w437) -> ()
                n242 = local write "cc"(w432) -> ()
                n243 = local write "baseline curv"(w438) -> ()
                n244 = local write "c_buffer 2"(w431) -> ()
              }
              frame #3 {
                w472 = 0.0 ("y")
                # "generate inputs for updating VRE"
                # "introduce momentum\nusing geometric sum"
                # "normalize \ngeometric sum"
                # "threshold to find active frames"
                n245 = local read "cc"() -> (w497:dbl)
                n246 = local read "zeroCross"() -> (w490:i16)
                n247 = local read "th2"() -> (w498:dbl)
                n248 = local read "m"() -> (w499:dbl)
                n249 = Divide(x=w497, y=20.0) -> (x/y=w458:dbl)
                n250 = Less Than 0?(x=w458) -> (x < 0?=w462:bool)
                n251 = Select(t=-1.0, s=w462, f=1.0) -> (s? t:f=w459:dbl)
                n252 = Compound Arithmetic op=MULTIPLY(w458, w458) -> (w463:dbl)
                n253 = Greater?(x=w499, y=w498) -> (0:w500:bool)
                n254 = Multiply(x=w463, y=w459) -> (x*y=w457:dbl)
                n255 = Boolean To (0,1)(Boolean=w500) -> (0, 1=w479:i16)
                n256 = Multiply(x=w457, y=w479) -> (x*y=w465:dbl)
                n257 = Multiply(x=w490, y=w479) -> (x*y=w487:i16)
                n258 = local read "decayR"() -> (w492:dbl)
                n259 = local read "decayF"() -> (w484:dbl)
                n260 = Multiply(x=w493, y=w492) -> (x*y=w496:dbl)
                n261 = Multiply(x=w488, y=w484) -> (x*y=w489:dbl)
                n262 = Add(x=w465, y=w496) -> (x+y=w491:dbl)
                n263 = Add(x=w487, y=w489) -> (x+y=w483:dbl)
                n264 = Replace Array Subset(array=w480, new element=w479, index=0) -> (w477:dbl[])
                n265 = Subtract(x=1.0, y=w492) -> (x-y=w494:dbl)
                n266 = Subtract(x=1.0, y=w484) -> (x-y=w486:dbl)
                n267 = Multiply(x=w491, y=w494) -> (x*y=w464:dbl)
                n268 = Multiply(x=w483, y=w486) -> (x*y=w469:dbl)
                n269 = local read "yawCoef_R"() -> (w475:dbl)
                n270 = local read "yawCoef_L"() -> (w476:dbl)
                n271 = local read "frdCoef"() -> (w473:dbl)
                n272 = Greater Or Equal To 0?(x=w464) -> (x >= 0?=w474:bool)
                n273 = Rotate 1D Array(1:w477, 2:1 ("n")) -> (0:w478:dbl[])
                n274 = Greater?(x=w473, y=w472) -> (0:w471:bool)
                n275 = case shown="True" w474 {
                  tunnel: w464 -> [w502 w506]
                  tunnel: [w503 w505] -> w467
                  tunnel: w475 -> [_ w504]
                  tunnel: w476 -> [w501 _]
                  frame False {
                    n276 = Multiply(x=w502, y=w501) -> (x*y=w503:dbl)
                  }
                  frame True {
                    n277 = Multiply(x=w506, y=w504) -> (x*y=w505:dbl)
                  }
                }
                "yaw display" <- w467
                n278 = Select(t=w473, s=w471, f=w472) -> (s? t:f=w470:dbl)
                n279 = Multiply(x=w469, y=w470) -> (x*y=→"forward display":dbl)
                n280 = local write "m_buffer2"(w477) -> ()
                n281 = local write "forward"(w469) -> ()
                n282 = local write "yaw"(w464) -> ()
                n283 = local write "yawInput"(w467) -> ()
              }
            }
            n284 = local read "loop time (ms)"() -> (w356:u32)
            n285 = Wait (ms)(milliseconds to wait=w356) -> ()  [unwired: 1 out]
            n286 = Tick Count (ms)() -> (millisecond timer value=w371:u32)
            n287 = Subtract(x=w371, y=w370) -> (x-y=w355:u32)
            n288 = local write "LV loop time"(w355) -> ()
            "i" <- w347
          }
        }
        frame True {
        }
      }
    }
    frame #4 {
      n289 = flat-sequence {
        frame #0 {
          n290 = local read "set 2P frames"() -> (w518:dbl)
          n291 = local read "2P fps"() -> (w522:dbl)
          n292 = local read "fileNumber"() -> (w513:string)
          n293 = Number To Decimal String(number=w522) -> (decimal integer string=w520:string)  [unwired: 1 in]
          n294 = Number To Decimal String(number=w518) -> (decimal integer string=w516:string)  [unwired: 1 in]
          n295 = Concatenate Strings("CONFIGURATION: enter 2P fps: ", w520, "\r", "MAIN CONTROLS: enter 2P frame number: ", w516, "\r", "enter 2P Acquisition number: ", w513, "\r", "Click EXT, then GRAB", "\r", "Receive message \"I m ready now!\"", "\r", "Click OK") -> (w523:string)
          n296 = call "Display Message to User"("Message"=w523) -> ()  [unwired: 9 in, 2 out]
        }
        frame #1 {
          # "trigger scanimageB"
          n297 = call "Convert to Dynamic Data"("Array"=dbl[] [5.0, 0.0]) -> ("Dynamic Data Type"=w524:dynamicdata)  [unwired: 3 in]
          n298 = call "DAQ Assistant2"("data"=w524) -> ()  [unwired: 17 in, 2 out]
        }
        frame #2 {
          n299 = Tick Count (ms)() -> (millisecond timer value=→"t0":u32)
        }
      }
    }
    frame #5 {
      # "length= 2*w"
      # "length= 2*w"
      # "length = w/2"
      # "length= w/2"
      n300 = local read "trackPt#"() -> (w533:i32)
      n301 = local read "txt row#"() -> (w532:u64)
      n302 = local read "txt row#"() -> (w547:u64)
      n303 = local read "Session Out"() -> (w539:T2)
      n304 = local read "m_buffer2"() -> (w528:i8[])
      n305 = local read "c_buffer 2"() -> (w529:dbl[])
      n306 = local read "m_buffer"() -> (w535:dbl[])
      n307 = local read "c_buffer"() -> (w536:dbl[])
      n308 = call "IMAQ Create"("Image Name"="roi") -> ("New Image"=w543:T1)  [unwired: 4 in, 1 out]
      n309 = call "IMAQ Create"("Image Name"="resample") -> ("New Image"=w541:T1)  [unwired: 4 in, 1 out]
      n310 = call "IMAQ Create"("Image Name"="raw") -> ("New Image"=w550:T1)  [unwired: 4 in, 1 out]
      n311 = Tick Count (ms)() -> (millisecond timer value=w540:u32)
      n312 = Initialize Array(0.0 ("element"), w547, 20 ("dimension size")) -> (w546:dbl[][])
      n313 = Initialize Array(0.0 ("element"), w532, w533) -> (w531:dbl[][])
      n314 = while {
        tunnel: w550 -> [w590]
        shift-right: [w587] -> w545
        shift-left: w546 -> [w588]
        shift-right: [w586] -> _
        shift-left: w540 -> [w585]
        tunnel: w543 -> [w584]
        tunnel: w541 -> [w583]
        tunnel: w539 -> [w577]
        shift-right: [w574] -> _
        shift-left: 0.0 -> [w575]
        shift-right: [w572] -> _
        shift-left: 0.0 -> [w573]
        shift-right: [w571] -> _
        shift-left: _ -> [w569]
        shift-right: [w570] -> _
        shift-left: _ -> [w567]
        shift-right: [w568] -> _
        shift-left: _ -> [w566]
        shift-right: [w563] -> _
        shift-left: w536 -> [w565]
        shift-right: [w562] -> _
        shift-left: w535 -> [w564]
        shift-right: [w560] -> w530
        shift-left: w531 -> [w561]
        shift-right: [w558] -> _
        shift-left: _ -> [w559]
        shift-right: [w556] -> _
        shift-left: w529 -> [w557]
        shift-right: [w554] -> _
        shift-left: w528 -> [w555]
        shift-right: [w553] -> _
        shift-left: 0.0 ("headingAngle") -> [w552]
        i -> [w578]
        stop <- w581 stop-if-true
        n315 = stacked-sequence {
          tunnel: w590 -> [_ _ _ w754 _ _ _ _ _ _ _ _]
          tunnel: w588 -> [_ _ _ _ _ _ _ _ _ _ w961 _]
          tunnel: [_ _ _ _ _ _ _ _ _ _ w960 _] -> w587
          tunnel: w584 -> [_ _ _ w752 _ _ _ _ _ _ _ _]
          tunnel: w583 -> [_ _ _ w753 _ _ _ _ _ _ _ _]
          tunnel: w578 -> [_ _ _ w746 _ _ _ _ _ _ w958 w969]
          tunnel: w577 -> [_ _ _ w755 _ _ _ _ _ _ _ _]
          tunnel: w575 -> [_ _ _ _ _ _ w843 _ _ _ _ _]
          tunnel: [_ _ _ _ _ _ w842 _ _ _ _ _] -> w574
          tunnel: w573 -> [_ _ _ _ _ _ _ w859 _ _ _ _]
          tunnel: [_ _ _ _ _ _ _ w857 _ _ _ _] -> w572
          tunnel: [_ _ _ _ w786 _ _ _ _ _ _ _] -> w571
          tunnel: [_ _ _ _ w790 _ _ _ _ _ _ _] -> w570
          tunnel: w569 -> [_ _ _ _ w790 _ _ _ _ _ _ _]
          tunnel: [_ _ _ _ w789 _ _ _ _ _ _ _] -> w568
          tunnel: w567 -> [_ _ _ _ w789 _ _ _ _ _ _ _]
          tunnel: w566 -> [_ _ _ _ w791 _ _ _ _ _ _ _]
          tunnel: w565 -> [_ _ _ _ w795 _ _ _ _ _ _ _]
          tunnel: w564 -> [_ _ _ _ w794 _ _ _ _ _ _ _]
          tunnel: [_ _ _ _ w792 _ _ _ _ _ _ _] -> w563
          tunnel: [_ _ _ _ w793 _ _ _ _ _ _ _] -> w562
          tunnel: w561 -> [_ _ _ w747 _ _ _ _ _ _ _ _]
          tunnel: [_ _ _ w749 _ _ _ _ _ _ _ _] -> w560
          tunnel: w559 -> [_ _ _ _ _ w813 _ _ _ _ _ _]
          tunnel: [_ _ _ _ _ w807 _ _ _ _ _ _] -> w558
          tunnel: w557 -> [_ _ _ _ _ w809 _ _ _ _ _ _]
          tunnel: [_ _ _ _ _ w808 _ _ _ _ _ _] -> w556
          tunnel: w555 -> [_ _ _ _ w777 _ _ _ _ _ _ _]
          tunnel: [_ _ _ _ w779 _ _ _ _ _ _ _] -> w554
          tunnel: [_ w620 _ _ _ _ _ _ _ _ _ _] -> w553
          tunnel: w552 -> [_ w622 _ _ _ _ _ _ _ _ _ _]
          frame #0 {
            # "update protocol parameters"
            n316 = flat-sequence {
              frame #0 {
                n317 = local read "t0"() -> (w612:u32)
                n318 = Tick Count (ms)() -> (millisecond timer value=w611:u32)
                n319 = Subtract(x=w611, y=w612) -> (x-y=w610:u32)
                n320 = local read "modDuration"() -> (w604:u16)
                n321 = Divide(x=w610, y=u32 1000) -> (x/y=w608:dbl)
                n322 = Round To Nearest(number=w608) -> (nearest integer value=w607:dbl)
                "expTime" <- w607
                n323 = Quotient & Remainder(x=w607, y=w604) -> (x-y*floor(x/y)=w602:dbl, floor(x/y)=w594:dbl)
                "moduleTime" <- w602
                n324 = local read "moviePrimedON"() -> (w603:u16)
                n325 = local read "moviePrimedOff"() -> (w601:u16)
                n326 = local read "perturbSeq"() -> (w595:u8[])
                n327 = local read "movieSeq"() -> (w596:u8[])
                n328 = Increment(x=w594) -> (x+1=→"moduleNum":dbl)
                n329 = Increment(x=w594) -> (x+1=w593:dbl)
                n330 = Greater Or Equal?(x=w602, y=w603) -> (x >= y?=w605:bool)
                n331 = Less?(x=w602, y=w601) -> (x < y?=w606:bool)
                n332 = Index Array(array=w596, index=w594) -> (element=→"movieID":u8)
                n333 = Index Array(array=w595, index=w594) -> (element=→"perturbID":u8)
                n334 = Index Array(array=w596, index=w593) -> (element=→"nextMovieID":u8)
                n335 = Index Array(array=w595, index=w593) -> (element=→"nextPerturbID":u8)
                n336 = And(x=w605, y=w606) -> (x .and. y?=→"moviePrimed":bool)
              }
              frame #1 {
                n337 = local read "moduleNumPrevious"() -> (w615:u8)
                n338 = local read "moduleNum"() -> (w616:u8)
                n339 = Subtract(x=w616, y=w615) -> (x-y=w614:u8)
                n340 = Not Equal To 0?(x=w614) -> (x != 0?=w613:bool)
                n341 = case shown="True" w613 {
                  frame False {
                  }
                  frame True {
                    w618 = 0 ("z1")
                    n342 = local read "movieID"() -> (w617:u8)
                    n343 = local write "z3"(w618) -> ()
                    n344 = local write "tON"(w618) -> ()
                    n345 = local write "z1"(w617) -> ()
                  }
                }
              }
              frame #2 {
                n346 = local read "moduleNum"() -> (→"moduleNumPrevious":u8)
              }
            }
          }
          frame #1 {
            # "0 (up), 270 (right) 180 (down), 90 (left)"
            # "headingAngle is unstable (flicker between HA and 0, causing problem in \"z3\" update)"
            # "update protocol parameters:"
            n347 = local read "headingAngle"() -> (w621:dbl)
            n348 = flat-sequence {
              tunnel: w620 -> [w631]
              frame #0 {
                # "z3 is a step function triggers the onset of movie presentation"
                n349 = local read "moviePrimed"() -> (w633:bool)
                n350 = local read "yawInput"() -> (w628:dbl)
                n351 = local read "Quiet mode"() -> (w630:bool)
                n352 = local read "z3"() -> (w636:u32)
                n353 = Less?(x=w631, y=20.0) -> (x < y?=w639:bool)
                n354 = Greater?(x=w631, y=340.0) -> (0:w638:bool)
                n355 = Equal To 0?(x=w636) -> (x = 0?=w634:bool)
                n356 = Or(x=w639, y=w638) -> (x .or. y?=w632:bool)
                n357 = Not(x=w630) -> (.not. x?=w629:bool)
                n358 = Less?(x=w628, y="yawIn threshold for movie") -> (x < y?=w626:bool)
                n359 = Compound Arithmetic op=AND(w629, w634, w633, w632, w626) -> (w635:bool)
                n360 = case shown="True" w635 {
                  frame False {
                  }
                  frame True {
                    n361 = local read "movieID"() -> (w642:u8)
                    n362 = local read "moduleTime"() -> (w641:u16)
                    n363 = local read "z3"() -> (w644:u32)
                    n364 = Increment(x=w644) -> (x+1=w645:u32)
                    n365 = Multiply(x=w645, y=w642) -> (x*y=w643:u32)
                    n366 = local write "tON"(w641) -> ()
                    n367 = local write "z3"(w643) -> ()
                  }
                }
              }
              frame #1 {
                # "Switch ON and OFF of VR halt and LR inversion"
                # "movieR records the duration of movie presentation, doesn't have a trigger function"
                n368 = local read "perturbDuration"() -> (w668:u16)
                n369 = local read "perturbOnset"() -> (w669:u16)
                n370 = local read "moduleTime"() -> (w666:u16)
                n371 = local read "moduleTime"() -> (w657:u16)
                n372 = local read "perturbID"() -> (w665:u8)
                n373 = local read "perturbID"() -> (w658:u8)
                n374 = local read "Quiet mode"() -> (w647:bool)
                n375 = local read "tON"() -> (w648:u16)
                n376 = Add(x=w669, y=w668) -> (x+y=w667:u16)
                n377 = Subtract(x=w657, y=w648) -> (x-y=w656:u16)
                n378 = Not Equal To 0?(x=w648) -> (x != 0?=w651:bool)
                n379 = Equal?(x=w665, y=u64 1) -> (x = y?=w663:bool)
                n380 = Equal?(x=w658, y=u64 2) -> (x = y?=w660:bool)
                n381 = Not(x=w647) -> (.not. x?=w646:bool)
                n382 = Greater?(x=w666, y=w669) -> (0:w654:bool)
                n383 = Less?(x=w666, y=w667) -> (x < y?=w653:bool)
                n384 = Less?(x=w656, y=36) -> (x < y?=w650:bool)
                n385 = And(x=w650, y=w651) -> (x .and. y?=w649:bool)
                n386 = Compound Arithmetic op=AND(w646, w654, w653) -> (→"perturb ON":bool)
                n387 = Compound Arithmetic op=AND(w646, w654, w653, w663) -> (w662:bool)
                n388 = Compound Arithmetic op=AND(w646, w654, w653, w660) -> (w661:bool)
                n389 = case shown="False" w662 {
                  frame False {
                    n390 = local write "hijack"(FALSE ("hijack")) -> ()
                  }
                  frame True {
                    n391 = local write "hijack"(TRUE ("hijack")) -> ()
                  }
                }
                n392 = case shown="True" w661 {
                  frame False {
                    n393 = local write "LR invert"(FALSE ("hijack")) -> ()
                  }
                  frame True {
                    n394 = local write "LR invert"(TRUE ("hijack")) -> ()
                  }
                }
                n395 = case shown="True" w649 {
                  frame False {
                    n396 = local write "movieR"(0 ("movieR")) -> ()
                  }
                  frame True {
                    n397 = local read "movieID"() -> (w671:u8)
                    n398 = local write "movieR"(w671) -> ()
                  }
                }
              }
              frame #2 {
                n399 = local read "movieR"() -> (w677:u8)
                n400 = Not Equal To 0?(x=w677) -> (x != 0?=→"movie ON":bool)
              }
            }
            n401 = Equal To 0?(x=w621) -> (x = 0?=w623:bool)
            n402 = case shown="False" w623 {
              tunnel: [w624 w625] -> w620
              tunnel: w622 -> [_ w625]
              tunnel: w621 -> [w624 _]
              frame False {
              }
              frame True {
              }
            }
          }
          frame #2 {
            # "Showing on the front panel when the next movie presentation and VR perturbation will occur"
            n403 = local read "perturbDuration"() -> (w710:u16)
            n404 = local read "moduleTime"() -> (w708:u16)
            n405 = local read "perturbOnset"() -> (w707:u16)
            n406 = local read "modDuration"() -> (w709:u16)
            n407 = local read "Quiet mode"() -> (w679:bool)
            n408 = Subtract(x=w709, y=w708) -> (x-y=w721:u16)
            n409 = Add(x=w707, y=w710) -> (x+y=w723:u16)
            n410 = Add(x=w721, y=w707) -> (x+y=w690:u16)
            n411 = Subtract(x=w707, y=w708) -> (x-y=w695:u16)
            n412 = Less?(x=w708, y=w707) -> (x < y?=w706:bool)
            n413 = Less?(x=w708, y=w723) -> (x < y?=w726:bool)
            n414 = Greater?(x=w708, y=w723) -> (0:w722:bool)
            n415 = Greater Or Equal?(x=w708, y=w707) -> (x >= y?=w725:bool)
            n416 = And(x=w725, y=w726) -> (x .and. y?=w724:bool)
            n417 = Select(t=u16 999, s=w679, f=w695) -> (s? t:f=w696:u16)
            n418 = Select(t=u16 999, s=w679, f=u16 0 ("nextPerturb")) -> (s? t:f=w688:u16)
            n419 = Select(t=u16 999, s=w679, f=w690) -> (s? t:f=w691:u16)
            n420 = case shown="True" w706 {
              tunnel: w696 -> [_ w738]
              frame False {
              }
              frame True {
                n421 = local read "perturbID"() -> (w737:u8)
                n422 = local write "perturb wait"(w738) -> ()
                n423 = local write "perturb"(w737) -> ()
              }
            }
            n424 = case shown="True" w724 {
              tunnel: w688 -> [_ w735]
              frame False {
              }
              frame True {
                n425 = local read "perturbID"() -> (w736:u8)
                n426 = local write "perturb wait"(w735) -> ()
                n427 = local write "perturb"(w736) -> ()
              }
            }
            n428 = case shown="True" w722 {
              tunnel: w691 -> [_ w734]
              frame False {
              }
              frame True {
                n429 = local read "nextPerturbID"() -> (w733:u8)
                n430 = local write "perturb wait"(w734) -> ()
                n431 = local write "perturb"(w733) -> ()
              }
            }
            n432 = local read "movieR"() -> (w701:u8)
            n433 = local read "moviePrimedON"() -> (w704:u16)
            n434 = local read "moviePrimedOff"() -> (w716:u16)
            n435 = local read "z3"() -> (w702:u32)
            n436 = local read "modDuration"() -> (w711:u16)
            n437 = local read "moduleTime"() -> (w703:u16)
            n438 = Equal To 0?(x=w701) -> (x = 0?=w699:bool)
            n439 = Not Equal To 0?(x=w702) -> (x != 0?=w700:bool)
            n440 = And(x=w699, y=w700) -> (x .and. y?=w698:bool)
            n441 = Subtract(x=w704, y=w703) -> (x-y=w685:u16)
            n442 = Greater Or Equal?(x=w703, y=w704) -> (x >= y?=w720:bool)
            n443 = Less?(x=w703, y=w716) -> (x < y?=w719:bool)
            n444 = Greater?(x=w703, y=w716) -> (0:w714:bool)
            n445 = Subtract(x=w711, y=w703) -> (x-y=w712:u16)
            n446 = Not(x=w698) -> (.not. x?=w697:bool)
            n447 = And(x=w720, y=w719) -> (x .and. y?=w717:bool)
            n448 = Less?(x=w703, y=w704) -> (x < y?=w705:bool)
            n449 = Add(x=w712, y=w704) -> (x+y=w680:u16)
            n450 = And(x=w717, y=w697) -> (x .and. y?=w718:bool)
            n451 = And(x=w717, y=w698) -> (x .and. y?=w713:bool)
            n452 = Or(x=w713, y=w714) -> (x .or. y?=w715:bool)
            n453 = Select(t=u16 999, s=w679, f=w685) -> (s? t:f=w686:u16)
            n454 = Select(t=u16 999, s=w679, f=u16 0 ("nextMovie")) -> (s? t:f=w682:u16)
            n455 = Select(t=u16 999, s=w679, f=w680) -> (s? t:f=w681:u16)
            n456 = case shown="True" w705 {
              tunnel: w686 -> [_ w732]
              frame False {
              }
              frame True {
                n457 = local read "movieID"() -> (w731:u8)
                n458 = local write "movie wait"(w732) -> ()
                n459 = local write "movie"(w731) -> ()
              }
            }
            n460 = case shown="True" w718 {
              tunnel: w682 -> [_ w729]
              frame False {
              }
              frame True {
                n461 = local read "movieID"() -> (w730:u8)
                n462 = local write "movie wait"(w729) -> ()
                n463 = local write "movie"(w730) -> ()
              }
            }
            n464 = case shown="True" w715 {
              tunnel: w681 -> [_ w728]
              frame False {
              }
              frame True {
                n465 = local read "nextMovieID"() -> (w727:u8)
                n466 = local write "movie wait"(w728) -> ()
                n467 = local write "movie"(w727) -> ()
              }
            }
          }
          frame #3 {
            # "tail tracking and calculate tail curvature"
            n468 = call <vilib>:"IMAQdx Grab.vi"("Image In"=w754, "Session In"=w755) -> ("Image Out"=w772:T1)  [unwired: 6 in, 3 out]
            n469 = local read "Xres"() -> (w766:i32)
            n470 = local read "Yres"() -> (w767:i32)
            n471 = call "IMAQ Resample"("X Resolution"=w766, "Y Resolution"=w767, "Image Dst"=w753, "Image Src"=w772) -> ("Image Dst Out"=w771:T1)  [unwired: 6 in, 1 out]
            n472 = local read "ROI"() -> (w773:i32[])
            n473 = call "IMAQ Extract 2"("Optional Rectangle"=w773, "Image Dst"=w752, "Image Src"=w771) -> ("Image Dst Out"=w740:T1)  [unwired: 7 in, 1 out]
            n474 = local read "th_darkBG"() -> (w759:dbl)
            n475 = local read "refine5ind"() -> (w762:dbl[])
            n476 = call "IMAQ ImageToArray"("Image"=w740) -> ("Image Pixels (U8)"=w745:u8[][])  [unwired: 3 in, 4 out]
            "I" <- w745
            n477 = local read "segL"() -> (w760:dbl)
            n478 = local read "qCtr"() -> (w761:dbl)
            n479 = local read "xc"() -> (w763:dbl)
            n480 = script code="im = double(I);\nbw = im>th;\nqq = bw;\nqq(1:segL,:)=0;\nif sum(qq(:))<qCtr, % <KH2016Jun> thresholded image should at least have this amount of pixel. If less, various error can occur during track point calculation.\n    bw = bwBackup;\nelse\n    bwBackup = bw;\nend\n% <KH2016Jun> only keep pixels connected by connectivity 4 (not 8).\n% This helps to remove fin pixels\n[L NUM] = bwlabeln(bw,4); % <KH2016Jun> I think you can also use regionprops as below\nR = zeros(1,NUM); % <KH2016Jun>\nfor k = 1:NUM, R(k) = sum(sum(L==k));end % <KH2016Jun>\nbw = bw.* L==find(R==max(R),1,'first'); % <KH2016Jun>\nim_ = bw.*im;\n\n% first tracking point\nPOIvalue = double(im_(1:3, xc-10:xc+10));\nx0 = sum(sum(repmat(xc-10:xc+10,3,1).*POIvalue))./sum(sum(POIvalue));\nif isnan(x0), x0 = round(fx/2); end % <KH2016Jun> Just to prevent error message show up later in the code.\ny0 = 2;\n\n% rest tracking points\nbw_ = bwmorph(bw,'thin',Inf);\n% rostral branches are complicated to clean, set rostral rows to zero\nbw_(1:segL,:)=0; % <KH2016Jun>\n% remove small segments, ex. head post, rostral branches\nlineStats = regionprops(bw_, {'Area','PixelIdxList'});\n[L, index] = max([lineStats.Area]);\nbw_ = bw_*0;\nbw_(lineStats(index).PixelIdxList) = 1;\n\nc = sum(bw_(:));\nind = find(bw_);\nPOI = repmat(refine5Ind,1,c)+repmat(ind',length(refine5Ind),1);\nif sum(sum(POI>(size(bw,1)*size(bw,2)) | POI<1))~= 0 % <KH2016Jun> In case POI is out of image range\n    POI = ones(size(POI));\nend\n\nPOIx = ceil(POI/fy);\nPOIy = rem(POI,fy);\nPOIvalue = double(im_(POI));\nx_ = sum(POIx.*POIvalue)./sum(POIvalue);\ny_ = sum(POIy.*POIvalue)./sum(POIvalue);\ntrackA = [x0, x_; y0, y_]; % non-sorted track points\n\nseed = [x0;y0];\nseedInd = 1;\ntrack_ = [zeros(2,1) trackA(:,2:end)]; % temporary registry\ntrack = trackA; % to store sorted track points\nfor j = 1:size(track,2)-1\n    d = ((track_(1,:)-seed(1)).^2 + (track_(2,:)-seed(2)).^2); % distance of all remaining points to the seed\n    targetInd = find(d==min(d),1,'first');\n    target = track_(:, targetInd);\n    track(:,j+1) = target;\n    seed = target;\n    track_(:,targetInd)=0;\nend\n\n% cut tail into 6 segments, (x0,y0)>(x1, y1) is seg 1. (x1, y1) > (xn, yn) is cut to 5 segments\nsegSize = (size(track,2)-2)/5; % an estimate of segment length (# of track point).\n% segSize is similar to segL, but it's more precise. IMP: do not try to replace with segL.\nt2 = track(:,round(2:segSize:size(track,2)));\nd2 = mean(sum(diff(t2,1,2).^2)); % an estimate of segment length (pixel distance)\ntrack_ = track(:,2:end-1); %<KH2016Jun>\nseed  = track_(:,1);\ntrack2 = [track(:,1:2) zeros(2,4) track(:,end)];\nfor j = 1:4\n    d = abs(((track_(1,:)-seed(1)).^2 + (track_(2,:)-seed(2)).^2)-d2);\n    targetInd = find(d==min(d),1,'first');\n    target = track_(:, targetInd);\n    track2(:,j+2) = target;\n    seed = target;\n    track_(:,1:targetInd)=0;\nend\n\ndV = diff(track2,[],2);\nAngle = atan(dV(1,:) ./ dV(2,:))/pi*180; % -90<angle<90\n% expand Angle from -90<angle<90 to -180<angle< 180\nAngle(dV(2,:)<0) = Angle(dV(2,:)<0) +180; %<KH2016Jun> -90<angle<270\nAngle(Angle>180) = Angle(Angle>180) -360; %<KH2016Jun> -180<angle<180\ncurv = diff(Angle);\n\ndd = sqrt(sum(diff(track2,1,2).^2));\nif sum(abs(curv)>60)==0 && sum(isnan(curv))==0 && sum(dd<segSize*0.5)==0%<KH2016Jun>\n    track2backup = track2;\n    curvBackup = curv;\nelse\n    if i==1;\n        track2 = [fx/2*ones(1,7);1:5:31]; % if first frame is bad, just set it as a vertical straight line\n        curv = zeros(1,5);\n    else\n        track2 = track2backup;\n        curv = curvBackup;\n    end\nend\n\ntrack2x = track2(1,:);\ntrack2y = track2(2,:);" ("Script Node")("I"=w745, "th"=w759, "segL"=w760, "qCtr"=w761, "refine5ind"=w762, "xc"=w763) -> ("track2x"=w751:dbl[], "track2y"=w750:dbl[], "curv"=w758:dbl[], "NUM"=w739:dbl)  [unwired: 1 in, 1 out]
            n481 = Decrement(x=w751) -> (x-1=w742:dbl[])
            n482 = Decrement(x=w750) -> (x-1=w741:dbl[])
            n483 = local write "blobs"(w739) -> ()
            n484 = for {
              tunnel: w742 -> [w776] mode=indexing
              tunnel: w741 -> [w775] mode=indexing
              tunnel: [w774] -> w743 mode=indexing
              n485 = Bundle(w776, w775) -> (w774:cluster{dbl, dbl})  [unwired: 1 in]
            }
            n486 = Array Size(array=w741) -> (size(s)=w765:i32)
            n487 = Array Subset(array=w758, index=2, length=3) -> (w768:dbl[])
            n488 = Multiply(x=w765, y=2) -> (x*y=w757:i32)
            n489 = Build Array (concatenate)(w742, w741) -> (w748:dbl[])
            n490 = call-poly <vilib>:"Mean.vi"("X"=w768) -> ("mean"=w756:dbl)  [unwired: 1 out]
            n491 = call "IMAQ Overlay Points"("Array of Points"=w743, "Image"=w740) -> ("Image Out"=→"Image_save":T1)  [unwired: 8 in, 1 out]
            n492 = Replace Array Subset(array=w747, new element=w748, index (row)=w746) -> (w749:dbl[][])  [unwired: 1 in]
            n493 = local write "trackPt#"(w757) -> ()
            n494 = local write "cCurv1"(w756) -> ()
          }
          frame #4 {
            # "threshold to find active frames"
            # "(1) update 2 sec buffers, \"c_buffer\" & \"m_buffers\" to calculate baseline curvature.\n(2) estimate tail movement \"m\"."
            n495 = local read "I"() -> (w786:u8[][])
            n496 = local read "cCurv1"() -> (w796:dbl)
            n497 = To Double Precision Float(number=w786) -> (double precision float=w803:dbl[][])
            n498 = To Double Precision Float(number=w791) -> (double precision float=w802:dbl[][])
            n499 = Subtract(x=w803, y=w802) -> (x-y=w806:dbl[][])
            n500 = Absolute Value(x=w806) -> (abs(x)=w805:dbl[][])
            n501 = local read "pix#"() -> (w801:i32)
            n502 = Add Array Elements(numeric array=w805) -> (sum=w804:dbl)
            n503 = Divide(x=w804, y=w801) -> (x/y=w781:dbl)
            n504 = local read "th2"() -> (w782:dbl)
            n505 = Greater?(x=w781, y=w782) -> (0:w785:bool)
            n506 = Boolean To (0,1)(Boolean=w785) -> (0, 1=w780:i16)
            "active" <- w780
            n507 = Replace Array Subset(array=w795, new element=w796, index=0) -> (w788:dbl[])
            "c_buffer" <- w788
            n508 = Replace Array Subset(array=w794, new element=w781, index=0) -> (w787:dbl[])
            "m_buffer" <- w787
            n509 = Replace Array Subset(array=w777, new element=w780, index=0) -> (w778:i8[])
            n510 = Rotate 1D Array(1:w788, 2:1 ("n")) -> (0:w792:dbl[])
            n511 = Rotate 1D Array(1:w787, 2:1 ("n")) -> (0:w793:dbl[])
            n512 = Rotate 1D Array(1:w778, 2:1 ("n")) -> (0:w779:i8[])
            n513 = local write "m"(w781) -> ()
            n514 = local write "m_buffer2"(w778) -> ()
          }
          frame #5 {
            # "avoid NaN when fish swim constantly, i.e. m_buffer always > th1"
            # "hijack baseline curvature"
            # "threshold to find inactive frames"
            n515 = local read "Set baseline curv = 0 (for debug)"() -> (w814:bool)
            n516 = local read "m_buffer"() -> (w827:dbl[])
            n517 = local read "c_buffer"() -> (w828:dbl[])
            n518 = local read "cCurv1"() -> (w826:dbl)
            n519 = local read "th1"() -> (w830:dbl)
            n520 = Less?(x=w827, y=w830) -> (x < y?=w831:bool[])
            n521 = Boolean To (0,1)(Boolean=w831) -> (0, 1=w833:i16[])
            n522 = Multiply(x=w828, y=w833) -> (x*y=w832:dbl[])
            n523 = Add Array Elements(numeric array=w832) -> (sum=w829:dbl)
            n524 = Add Array Elements(numeric array=w833) -> (sum=w819:i16)
            n525 = Divide(x=w829, y=w819) -> (x/y=w820:dbl)
            n526 = Greater?(x=w819, y=10.0) -> (0:w822:bool)
            n527 = Select(t=w820, s=w822, f=0.0) -> (s? t:f=w824:dbl)
            n528 = Select(t=0.0, s=w814, f=w824) -> (s? t:f=w816:dbl)
            n529 = Subtract(x=w826, y=w816) -> (x-y=w807:dbl)
            n530 = Replace Array Subset(array=w809, new element=w807, index=0) -> (w810:dbl[])
            n531 = Multiply(x=w813, y=w807) -> (x*y=w817:dbl)
            n532 = Less Than 0?(x=w817) -> (x < 0?=w818:bool)
            n533 = Boolean To (0,1)(Boolean=w818) -> (0, 1=w815:i16)
            n534 = Rotate 1D Array(1:w810, 2:1 ("n")) -> (0:w808:dbl[])
            n535 = local write "c_buffer 2"(w810) -> ()
            n536 = local write "zeroCross"(w815) -> ()
            n537 = local write "cc"(w807) -> ()
            n538 = local write "baseline curv"(w816) -> ()
          }
          frame #6 {
            # "Normalize the geometric sum\nso that a constant cc = K generates \nyaw = K."
            # "Introduce an exponential decay \nafter a pulse response."
            # "generate yaw input to VRE"
            n539 = local read "cc"() -> (w839:dbl)
            n540 = Divide(x=w839, y=20.0) -> (x/y=w837:dbl)
            n541 = case shown="True" "cc^2" {
              tunnel: w837 -> [w848 w850]
              tunnel: [w848 w849] -> w836
              frame False {
              }
              frame True {
                n542 = Less Than 0?(x=w850) -> (x < 0?=w854:bool)
                n543 = Select(t=-1.0, s=w854, f=1.0) -> (s? t:f=w851:dbl)
                n544 = Compound Arithmetic op=MULTIPLY(w850, w850) -> (w855:dbl)
                n545 = Multiply(x=w855, y=w851) -> (x*y=w849:dbl)
              }
            }
            n546 = local read "active"() -> (w841:i16)
            n547 = local read "decayR"() -> (w844:dbl)
            n548 = Multiply(x=w836, y=w841) -> (x*y=w838:dbl)
            n549 = Multiply(x=w843, y=w844) -> (x*y=w847:dbl)
            n550 = Add(x=w838, y=w847) -> (x+y=w842:dbl)
            n551 = Subtract(x=1.0, y=w844) -> (x-y=w845:dbl)
            n552 = Multiply(x=w842, y=w845) -> (x*y=w834:dbl)
            n553 = local write "yaw"(w834) -> ()
          }
          frame #7 {
            # "Introduce an exponential decay \nafter a pulse response."
            # "Normalize the geometric sum\nso that a constant cc = K generates \nyaw = K."
            # "generate foward input to VRE"
            n554 = local read "zeroCross"() -> (w858:i16)
            n555 = local read "active"() -> (w856:i16)
            n556 = Multiply(x=w858, y=w856) -> (x*y=w864:i16)
            n557 = local read "decayF"() -> (w861:dbl)
            n558 = Multiply(x=w859, y=w861) -> (x*y=w865:dbl)
            n559 = Add(x=w864, y=w865) -> (x+y=w857:dbl)
            n560 = Subtract(x=1.0, y=w861) -> (x-y=w863:dbl)
            n561 = Multiply(x=w857, y=w863) -> (x*y=w860:dbl)
            n562 = local write "forward"(w860) -> ()
          }
          frame #8 {
            # "Indroduce hijack mode to allow user control of VRE"
            # "VRE (HA_) rotates clockwise\nLabview XY plot rotates CCW"
            # "communicate with Python using COM"
            # "Display virtual position \nand heading direction"
            # "crosstalk between labview and python (Panda3D)\nsend: yawInput, forwadInput, movieID to Panda\nreceive: virtual position, heading direction.\nLabPythonRESET.vi is set to highest execution priority"
            n563 = case shown="True" "hijack" {
              tunnel: [w905 w919] -> w869
              tunnel: [w907 w915] -> w870
              tunnel: [FALSE ("reset_") "frdOmrVRE"] -> w871
              frame False {
                w898 = 0.0 ("y")
                n564 = local read "yaw"() -> (w896:dbl)
                n565 = local read "forward"() -> (w901:dbl)
                n566 = Greater Or Equal To 0?(x=w896) -> (x >= 0?=w904:bool)
                n567 = Greater?(x="frdCoef", y=w898) -> (0:w900:bool)
                n568 = case shown="False" w904 {
                  tunnel: w896 -> [w909 w913]
                  tunnel: [w910 w912] -> w905
                  tunnel: "yawCoef_R" -> [_ w911]
                  tunnel: "yawCoef_L" -> [w908 _]
                  frame False {
                    n569 = Multiply(x=w909, y=w908) -> (x*y=w910:dbl)
                  }
                  frame True {
                    n570 = Multiply(x=w913, y=w911) -> (x*y=w912:dbl)
                  }
                }
                n571 = Select(t="frdCoef", s=w900, f=w898) -> (s? t:f=w897:dbl)
                n572 = Multiply(x=w901, y=w897) -> (x*y=w907:dbl)
              }
              frame True {
                n573 = Divide(x="yaw_hijack", y="hijCoef1") -> (x/y=w919:dbl)
                n574 = Divide(x="frd_hijack", y="hijCoef2") -> (x/y=w915:dbl)
              }
            }
            n575 = Or(x="LR invert", y="LR invert manual") -> (x .or. y?=w866:bool)
            "LR invert all" <- w866
            n576 = local read "z3"() -> (w876:u32)
            n577 = local read "z1"() -> (w875:u32)
            n578 = Select(t=-1.0, s=w866, f=1.0) -> (s? t:f=w888:dbl)
            n579 = Add(x=w870, y="frdDrift") -> (x+y=w874:dbl)
            "frdInput" <- w874
            n580 = Multiply(x=w888, y=w869) -> (x*y=w889:dbl)
            n581 = Add(x="yawDrift", y=w889) -> (x+y=w873:dbl)
            "yawInput" <- w873
            n582 = call "LabviewPython_reset.vi"("frdOmr_"=w871, "reset_"=FALSE, "movie L"=w876, "movie R"=w875, "forward_"=w874, "yaw_"=w873) -> ("vreFps"=→"vreFps (ms)":dbl, "HA_"=w881:dbl, "y_"=w882:dbl, "x_"=w883:dbl)  [unwired: 2 in]
            "y" <- w882
            n583 = Negate(x=w881) -> (-x=w893:dbl)
            n584 = Not Equal To 0?(x=w883) -> (x != 0?=w878:bool)
            n585 = Not Equal To 0?(x=w882) -> (x != 0?=w879:bool)
            n586 = Not Equal To 0?(x=w881) -> (x != 0?=w880:bool)
            n587 = Negate(x=w883) -> (-x=w886:dbl)
            "x" <- w886
            n588 = Compound Arithmetic op=AND(w878, w879, w880) -> (w877:bool)
            n589 = Quotient & Remainder(x=w893, y=360.0) -> (x-y*floor(x/y)=w885:dbl)  [unwired: 1 out]
            "headingAngle" <- w885
            n590 = case shown="True" w877 {
              tunnel: w885 -> [_ w923]
              tunnel: w882 -> [_ w922]
              tunnel: w886 -> [_ w921]
              frame False {
              }
              frame True {
                n591 = call "simple fish4.vi"("pointer length"=30.0, "orientation"=w923, "y"=w922, "x"=w921) -> ("XY Graph"=→"virtual location":cluster{dbl[], dbl[]}[])  [unwired: 7 in]
              }
            }
            n592 = local write "yaw display"(w873) -> ()
            n593 = local write "forward display"(w874) -> ()
          }
          frame #9 {
            w930 = 660.0 ("y")
            w929 = 8000.0 ("y")
            # "In 2P data, every 8K framesare saved as a single tiff file.\nFor simplicity of data analysis, avoid introducing perturbations \nacross two tiff files."
            # "dev2/ctr2"
            # "read  the current frame number in scanimageB"
            n594 = call "DAQ Assistant"() -> ("data"=w935:dynamicdata)  [unwired: 16 in, 3 out]
            n595 = call "Convert from Dynamic Data"("Dynamic Data Type"=w935) -> ("Array"=w934:dbl[])  [unwired: 3 in]
            n596 = Index Array(array=w934) -> (element=w933:dbl)  [unwired: 1 in]
            "2P frame" <- w933
            n597 = Quotient & Remainder(x=w933, y=w929) -> (x-y*floor(x/y)=w927:dbl)  [unwired: 1 out]
            n598 = Subtract(x=w929, y=w930) -> (x-y=w928:dbl)
            n599 = Less?(x=w927, y=w930) -> (x < y?=w931:bool)
            n600 = Greater?(x=w927, y=w928) -> (0:w932:bool)
            n601 = Or(x=w931, y=w932) -> (x .or. y?=→"Don't":bool)
          }
          frame #10 {
            # "collect dynamic data (.txt)"
            n602 = local read "LR invert all"() -> (w936:bool)
            n603 = local read "headingAngle"() -> (w952:dbl)
            n604 = local read "baseline curv"() -> (w943:dbl)
            n605 = local read "LV loop time"() -> (w955:u32)
            n606 = local read "yawCoef_R"() -> (w940:dbl)
            n607 = local read "hijack"() -> (w957:bool)
            n608 = local read "vreFps (ms)"() -> (w951:dbl)
            n609 = local read "yawCoef_L"() -> (w939:dbl)
            n610 = local read "2P frame"() -> (w942:dbl)
            n611 = local read "frdCoef"() -> (w938:dbl)
            n612 = local read "yawInput"() -> (w948:dbl)
            n613 = local read "yawDrift"() -> (w946:dbl)
            n614 = local read "frdDrift"() -> (w941:dbl)
            n615 = local read "frdInput"() -> (w949:dbl)
            n616 = local read "movieR"() -> (w956:u8)
            n617 = local read "cCurv1"() -> (w944:dbl)
            n618 = local read "m"() -> (w945:dbl)
            n619 = Boolean To (0,1)(Boolean=w957) -> (0, 1=w950:i16)
            n620 = local read "y"() -> (w953:dbl)
            n621 = local read "x"() -> (w954:dbl)
            n622 = Boolean To (0,1)(Boolean=w936) -> (0, 1=w947:i16)
            n623 = Build Array(w948, w949, w950, w956, 0.0 ("element"), w955, w954, w953, w952, w951, w947, w946, w945, w944, w943, w942, w941, w940, w939, w938) -> (w959:dbl[])
            n624 = Replace Array Subset(array=w961, new element=w959, index (row)=w958) -> (w960:dbl[][])  [unwired: 1 in]
          }
          frame #11 {
            # "save tiff"
            n625 = local read "Image_save"() -> (w971:T1)
            n626 = local read "data tif"() -> (w972:refnum<file>)
            n627 = local read "txt row#"() -> (w970:u64)
            n628 = Subtract(x=w970, y=w969) -> (x-y=w967:u64)
            n629 = call "IMAQ ImageToArray"("Image"=w971) -> ("Image Pixels (U8)"=w978:u8[][])  [unwired: 3 in, 4 out]
            n630 = call "IMAQ GetImageSize"("Image"=w971) -> ("Y Resolution"=w977:i32, "X Resolution"=w976:i32)  [unwired: 3 in, 1 out]
            n631 = Multiply(x=w976, y=w977) -> (x*y=w975:i32)
            n632 = local read "loop time (ms)"() -> (w968:u32)
            n633 = Reshape Array(w978, w975) -> (w974:u8[])
            n634 = Write to Binary File(file (use dialog)=w972, data=w974, 5:FALSE ("prepend array or string size? (T)")) -> ()  [unwired: 3 in, 3 out]
            n635 = Compound Arithmetic op=MULTIPLY(w968, w967, 0.001) -> (w965:dbl)
            n636 = Quotient & Remainder(x=w965, y=60.0) -> (x-y*floor(x/y)=→"sec":dbl, floor(x/y)=→"min":dbl)
          }
        }
        n637 = Wait (ms)(milliseconds to wait="loop time (ms)") -> ()  [unwired: 1 out]
        n638 = Tick Count (ms)() -> (millisecond timer value=w586:u32)
        n639 = Subtract(x=w586, y=w585) -> (x-y=→"LV loop time":u32)
        n640 = local read "txt row#"() -> (w582:u64)
        n641 = Equal?(x=w578, y=w582) -> (x = y?=w579:bool)
        n642 = Or(x="forced stop", y=w579) -> (x .or. y?=w581:bool)
      }
      "txt" <- w545
      "trackPt" <- w530
    }
    frame #6 {
      # "dynamic parameters"
      # "const. parameters"
      n643 = local read "trackPt txt"() -> (w1008:path)
      n644 = local read "trackPt"() -> (w1007:dbl[][])
      n645 = Build Array("setLVloopT", "decayR", "decayF", "th1", "th2", "thBG", "modDur", "pertON", "pertDur", "movPrOn", "movPrOff") -> (w979:string[])
      n646 = local read "moviePrimedON"() -> (w986:u16)
      n647 = Build Array("yawIn", "frdIn", "hijack", "movieR", "movieL", "LVloop", "X", "Y", "HA", "VREloop", "LRinv.", "yawDrif", "movem", "cCurv1", "bCurv", "2Pflag", "frdDrif", "yawCoR", "yawCoL", "frdCo") -> (w1016:string[])
      n648 = local read "moviePrimedOff"() -> (w985:u16)
      n649 = local read "perturbDuration"() -> (w987:u16)
      n650 = local read "loop time (ms)"() -> (w1014:u32)
      n651 = local read "modDuration"() -> (w989:u16)
      n652 = local read "perturbOnset"() -> (w988:u16)
      n653 = local read "th_darkBG"() -> (w994:dbl)
      n654 = local read "decayR"() -> (w1012:dbl)
      n655 = local read "decayF"() -> (w997:dbl)
      n656 = local read "th1"() -> (w999:dbl)
      n657 = local read "th2"() -> (w998:dbl)
      n658 = Build Array(w1014, w1012, w997, w999, w998, w994, w989, w988, w987, w986, w985) -> (w1028:dbl[])
      n659 = local read "txt"() -> (w1030:dbl[][])
      n660 = Number To Fractional String(number=w1028, precision (6)=i16 1) -> (F-format string=w1027:string[])  [unwired: 2 in]
      n661 = Number To Fractional String(number=w1030, precision (6)=i16 3) -> (F-format string=w1033:string[][])  [unwired: 2 in]
      n662 = Build Array(w979, w1027) -> (w1026:string[][])
      n663 = Build Array (concatenate)(w1016, w1033) -> (w1032:string[][])
      n664 = local read "par txt"() -> (w1035:path)
      n665 = local read "data txt"() -> (w1031:path)
      n666 = call-poly <vilib>:"Write To Spreadsheet File.vi"("2D data"=w1007, "file path (dialog if empty)"=w1008) -> ()  [unwired: 6 in, 1 out]
      n667 = call-poly <vilib>:"Write To Spreadsheet File.vi"("transpose? (no:F)"=TRUE, "2D data"=w1026, "file path (dialog if empty)"=w1035) -> ()  [unwired: 5 in, 1 out]
      n668 = call-poly <vilib>:"Write To Spreadsheet File.vi"("2D data"=w1032, "file path (dialog if empty)"=w1031) -> ()  [unwired: 6 in, 1 out]
    }
    frame #7 {
      w1037 = 0.0 ("yaw_")
      n669 = local read "Session Out"() -> (w1039:T2)
      n670 = call "IMAQ Dispose"("All Images? (No)"=TRUE) -> ()  [unwired: 5 in, 1 out]
      n671 = call <vilib>:"IMAQdx Close Camera.vi"("Session In"=w1039) -> ()  [unwired: 10 in, 1 out]
      n672 = call "LabviewPython_reset.vi"("reset_"=TRUE, "movie L"=w1037, "movie R"=w1037, "forward_"=w1037, "yaw_"=w1037) -> ()  [unwired: 3 in, 4 out]
    }
  }
